vi "Auto.vi"() -> ()   [LabVIEW 2020]
uses:
  Global_Variable/A180648.vi
  Global_Variable/Global.vi
  Global_Variable/System_Conf.vi
  <userlib>/_MGI/1D Array/MGI Running Average/MGI Running Average(SGL).vi
  <userlib>/_MGI/1D Array/MGI Running Average/MGI Running Average(DBL).vi
  Libraries/S7/S7.lvlib
panel:
  out "磨合正向初始化":bool
  out "磨合逆向初始化":bool
  out "试验项_Event":refnum<user-event>
  out "产品_EVENT":refnum<user-event>
  out "布尔":bool=TRUE
  out "T1+T2":dbl
  out "T2":dbl
  out "T1":dbl
  out "吸收电流":sgl
  out "输出扭矩(大)":sgl
  out "输入扭矩":sgl
  out "力特性逆向去程":bool
  out "力特性正向去程":bool
  out "力特性逆向回程":bool
  out "力特性正向回程":bool
  out "逆向空载正向初始化":bool
  out "逆向空载逆向初始化":bool
  out "功能正向初始化":bool
  out "功能逆向初始化":bool
  out "空载逆向初始化":bool
  out "空载正向初始化":bool
  out "当前车速":i32
  out "试验项目":T1(tab)
  out "空载试验":cluster{dbl[], dbl[]}[](graph)
  out "功能试验":cluster{dbl[], dbl[]}[](graph)
  out "力特性试验":cluster{dbl[], dbl[]}[](graph)
  out "电流特性试验":cluster{dbl[], dbl[]}[](graph)
  out "传感器特性试验":cluster{dbl[], dbl[]}[](graph)
  out "逆向空载试验":cluster{dbl[], dbl[]}[](graph)
  out "磨合":cluster{dbl[], dbl[]}[](graph)
  out "振动2NHV-FFT":cluster{"f0":dbl, "df":dbl, "magnitude":dbl[]}[](graph)
  out "振动1NVH-FFT":cluster{"f0":dbl, "df":dbl, "magnitude":dbl[]}[](graph)
  in  "判定结果":bool[][](array[boolean])=[[TRUE]]
  in  "STEP":string
  # "车速0"
  # "车速1"
  # "车速2"
  # "车速3"
  # "车速4"
  # "车速5"
  # "车速0"
  # "车速1"
  # "车速2"
  # "车速3"
  # "车速4"
  # "车速5"
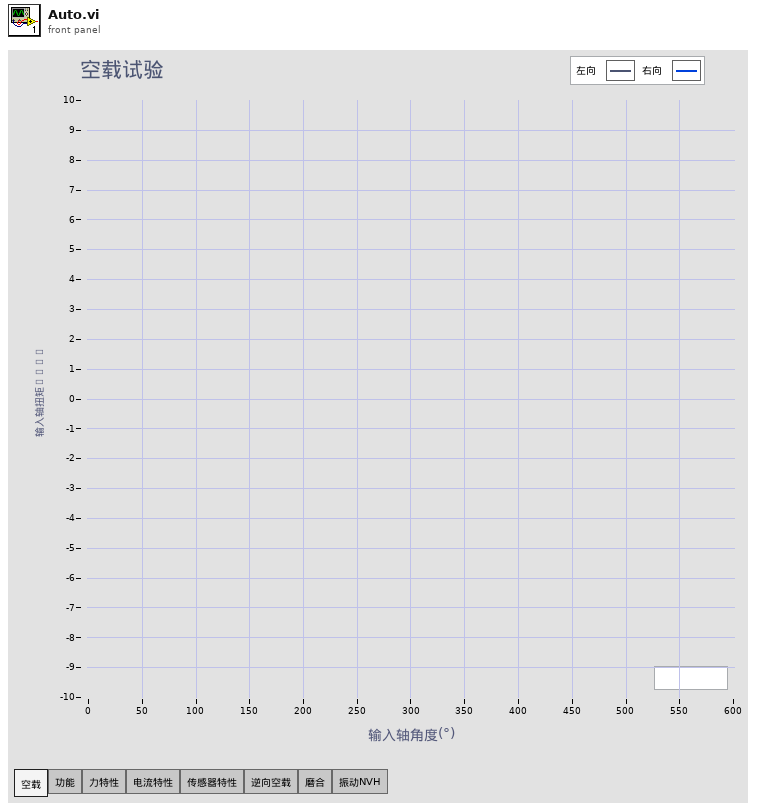
[diagram p1: front panel]
types:
  T1 = enum32{"空载", "功能", "力特性", "电流特性", "传感器特性", "逆向空载", "磨合", "振动NVH"}
  T2 = enum32{"Invalid", "Standard", "Closed", "Hidden", "Minimized", "Maximized"}
  T3 = cluster{"输入轴扭矩":dbl, "输出轴扭矩小量程":dbl, "输出轴扭矩大量程":dbl}
  T4 = enum32{"空载", "功能", "力特性", "电流特性", "传感器特性", "逆向空载", "振动NVH", "磨合", "完成"}
  T5 = enum16{"Left Button", "Center Button", "Right Button", "Window Close"}
  T6 = enum16{"角度标定状态", "角度标定", "角度标定清除", "扭矩标定状态", "扭矩标定", "扭矩标定清除", "内部软件版本号", "客户软件版本号"}
  T7 = typedef "System_conf.ctl" = cluster{"空载滤波":bool, "逆向空载滤波":bool, "空载扭矩系数":dbl, "逆向空载扭矩系数":dbl}
  T8 = enum32{"Bad", "Idle", "Run top level", "Running"}
  T9 = cluster{"扭矩判定范围":cluster{"单位":string, "下限":dbl, "上限":dbl}, "正向扭矩最大值":cluster{"单位":string, "下限":dbl, "上限":dbl}, "正向扭矩最小值":cluster{"单位":string, "下限":dbl, "上限":dbl}, "正向扭矩平均值":cluster{"单位":string, "下限":dbl, "上限":dbl}, "正向扭矩波动值":cluster{"单位":string, "下限":dbl, "上限":dbl}, "逆向扭矩最大值":cluster{"单位":string, "下限":dbl, "上限":dbl}, "逆向扭矩最小值":cluster{"单位":string, "下限":dbl, "上限":dbl}, "逆向扭矩平均值":cluster{"单位":string, "下限":dbl, "上限":dbl}, "逆向扭矩波动值":cluster{"单位":string, "下限":dbl, "上限":dbl}, "正逆向扭矩差值":cluster{"单位":string, "下限":dbl, "上限":dbl}, "启动力矩":cluster{"单位":string, "下限":dbl, "上限":dbl}}
  T10 = cluster{"扭矩判定范围":cluster{"单位":string, "下限":dbl, "上限":dbl}, "正向扭矩最大值":cluster{"单位":string, "下限":dbl, "上限":dbl}, "正向扭矩最小值":cluster{"单位":string, "下限":dbl, "上限":dbl}, "正向扭矩平均值":cluster{"单位":string, "下限":dbl, "上限":dbl}, "正向扭矩波动值":cluster{"单位":string, "下限":dbl, "上限":dbl}, "逆向扭矩最大值":cluster{"单位":string, "下限":dbl, "上限":dbl}, "逆向扭矩最小值":cluster{"单位":string, "下限":dbl, "上限":dbl}, "逆向扭矩平均值":cluster{"单位":string, "下限":dbl, "上限":dbl}, "逆向扭矩波动值":cluster{"单位":string, "下限":dbl, "上限":dbl}, "正逆向扭矩差值":cluster{"单位":string, "下限":dbl, "上限":dbl}}
  T11 = cluster{"对称性检测点":cluster{"单位":string, "下限":dbl, "上限":dbl}, "对称度":cluster{"单位":string, "下限":dbl, "上限":dbl}, "目标输出扭矩1":cluster{"单位":string, "下限":dbl, "上限":dbl}, "目标1正向输入扭矩":cluster{"单位":string, "下限":dbl, "上限":dbl}, "目标1逆向输入扭矩":cluster{"单位":string, "下限":dbl, "上限":dbl}, "目标1正逆向扭矩差":cluster{"单位":string, "下限":dbl, "上限":dbl}, "目标1输入扭矩滞后":cluster{"单位":string, "下限":dbl, "上限":dbl}, "目标输出扭矩2":cluster{"单位":string, "下限":dbl, "上限":dbl}, "目标2正向输入扭矩":cluster{"单位":string, "下限":dbl, "上限":dbl}, "目标2逆向输入扭矩":cluster{"单位":string, "下限":dbl, "上限":dbl}, "目标2正逆向扭矩差":cluster{"单位":string, "下限":dbl, "上限":dbl}, "目标2输入扭矩滞后":cluster{"单位":string, "下限":dbl, "上限":dbl}, "目标输出扭矩3":cluster{"单位":string, "下限":dbl, "上限":dbl}, "目标3正向输入扭矩":cluster{"单位":string, "下限":dbl, "上限":dbl}, "目标3逆向输入扭矩":cluster{"单位":string, "下限":dbl, "上限":dbl}, "目标3正逆向扭矩差":cluster{"单位":string, "下限":dbl, "上限":dbl}, "目标3输入扭矩滞后":cluster{"单位":string, "下限":dbl, "上限":dbl}, "目标输出扭矩4":cluster{"单位":string, "下限":dbl, "上限":dbl}, "目标4正向输入扭矩":cluster{"单位":string, "下限":dbl, "上限":dbl}, "目标4逆向输入扭矩":cluster{"单位":string, "下限":dbl, "上限":dbl}, "目标4正逆向扭矩差":cluster{"单位":string, "下限":dbl, "上限":dbl}, "目标4输入扭矩滞后":cluster{"单位":string, "下限":dbl, "上限":dbl}, "目标输出扭矩5":cluster{"单位":string, "下限":dbl, "上限":dbl}, "目标5正向输入扭矩":cluster{"单位":string, "下限":dbl, "上限":dbl}, "目标5逆向输入扭矩":cluster{"单位":string, "下限":dbl, "上限":dbl}, "目标5正逆向扭矩差":cluster{"单位":string, "下限":dbl, "上限":dbl}, "目标5输入扭矩滞后":cluster{"单位":string, "下限":dbl, "上限":dbl}}[]
  T12 = cluster{"主副信号和MAX":cluster{"单位":string, "下限":dbl, "上限":dbl}, "主副信号和MIN":cluster{"单位":string, "下限":dbl, "上限":dbl}, "主信号线性误差":cluster{"单位":string, "下限":dbl, "上限":dbl}, "副信号线性误差":cluster{"单位":string, "下限":dbl, "上限":dbl}, "主信号MAX":cluster{"单位":string, "下限":dbl, "上限":dbl}, "主信号MIN":cluster{"单位":string, "下限":dbl, "上限":dbl}, "副信号MAX":cluster{"单位":string, "下限":dbl, "上限":dbl}, "副信号MIN":cluster{"单位":string, "下限":dbl, "上限":dbl}, "中心偏移量":cluster{"单位":string, "下限":dbl, "上限":dbl}, "定点设置":cluster{"单位":string, "下限":dbl, "上限":dbl}, "定点左侧主信号":cluster{"单位":string, "下限":dbl, "上限":dbl}, "定点左侧副信号":cluster{"单位":string, "下限":dbl, "上限":dbl}, "定点右侧主信号":cluster{"单位":string, "下限":dbl, "上限":dbl}, "定点右侧副信号":cluster{"单位":string, "下限":dbl, "上限":dbl}}
  T13 = cluster{"对称性检测点":cluster{"单位":string, "下限":dbl, "上限":dbl}, "对称度":cluster{"单位":string, "下限":dbl, "上限":dbl}, "最大电流":cluster{"单位":string, "下限":dbl, "上限":dbl}, "目标输出电流1":cluster{"单位":string, "下限":dbl, "上限":dbl}, "目标1正向输入扭矩":cluster{"单位":string, "下限":dbl, "上限":dbl}, "目标1逆向输入扭矩":cluster{"单位":string, "下限":dbl, "上限":dbl}, "目标1正逆向扭矩差":cluster{"单位":string, "下限":dbl, "上限":dbl}, "目标1输入扭矩滞后":cluster{"单位":string, "下限":dbl, "上限":dbl}, "目标输出电流2":cluster{"单位":string, "下限":dbl, "上限":dbl}, "目标2正向输入扭矩":cluster{"单位":string, "下限":dbl, "上限":dbl}, "目标2逆向输入扭矩":cluster{"单位":string, "下限":dbl, "上限":dbl}, "目标2正逆向扭矩差":cluster{"单位":string, "下限":dbl, "上限":dbl}, "目标2输入扭矩滞后":cluster{"单位":string, "下限":dbl, "上限":dbl}, "目标输出电流3":cluster{"单位":string, "下限":dbl, "上限":dbl}, "目标3正向输入扭矩":cluster{"单位":string, "下限":dbl, "上限":dbl}, "目标3逆向输入扭矩":cluster{"单位":string, "下限":dbl, "上限":dbl}, "目标3正逆向扭矩差":cluster{"单位":string, "下限":dbl, "上限":dbl}, "目标3输入扭矩滞后":cluster{"单位":string, "下限":dbl, "上限":dbl}, "目标输出电流4":cluster{"单位":string, "下限":dbl, "上限":dbl}, "目标4正向输入扭矩":cluster{"单位":string, "下限":dbl, "上限":dbl}, "目标4逆向输入扭矩":cluster{"单位":string, "下限":dbl, "上限":dbl}, "目标4正逆向扭矩差":cluster{"单位":string, "下限":dbl, "上限":dbl}, "目标4输入扭矩滞后":cluster{"单位":string, "下限":dbl, "上限":dbl}, "目标输出电流5":cluster{"单位":string, "下限":dbl, "上限":dbl}, "目标5正向输入扭矩":cluster{"单位":string, "下限":dbl, "上限":dbl}, "目标5逆向输入扭矩":cluster{"单位":string, "下限":dbl, "上限":dbl}, "目标5正逆向扭矩差":cluster{"单位":string, "下限":dbl, "上限":dbl}, "目标5输入扭矩滞后":cluster{"单位":string, "下限":dbl, "上限":dbl}}[]
  T14 = cluster{"振动1频率检测段1范围":cluster{"单位":string, "下限":dbl, "上限":dbl}, "振动1频率检测段2范围":cluster{"单位":string, "下限":dbl, "上限":dbl}, "振动1频率检测段3范围":cluster{"单位":string, "下限":dbl, "上限":dbl}, "振动1频率检测段4范围":cluster{"单位":string, "下限":dbl, "上限":dbl}, "振动1频率检测段5范围":cluster{"单位":string, "下限":dbl, "上限":dbl}, "振动2频率检测段1范围":cluster{"单位":string, "下限":dbl, "上限":dbl}, "振动2频率检测段2范围":cluster{"单位":string, "下限":dbl, "上限":dbl}, "振动2频率检测段3范围":cluster{"单位":string, "下限":dbl, "上限":dbl}, "振动2频率检测段4范围":cluster{"单位":string, "下限":dbl, "上限":dbl}, "振动2频率检测段5范围":cluster{"单位":string, "下限":dbl, "上限":dbl}}
  T15 = cluster{"振动1频率检测段1振幅":cluster{"单位":string, "下限":dbl, "上限":dbl}, "振动1频率检测段2振幅":cluster{"单位":string, "下限":dbl, "上限":dbl}, "振动1频率检测段3振幅":cluster{"单位":string, "下限":dbl, "上限":dbl}, "振动1频率检测段4振幅":cluster{"单位":string, "下限":dbl, "上限":dbl}, "振动1频率检测段5振幅":cluster{"单位":string, "下限":dbl, "上限":dbl}, "振动2频率检测段1振幅":cluster{"单位":string, "下限":dbl, "上限":dbl}, "振动2频率检测段2振幅":cluster{"单位":string, "下限":dbl, "上限":dbl}, "振动2频率检测段3振幅":cluster{"单位":string, "下限":dbl, "上限":dbl}, "振动2频率检测段4振幅":cluster{"单位":string, "下限":dbl, "上限":dbl}, "振动2频率检测段5振幅":cluster{"单位":string, "下限":dbl, "上限":dbl}}
  T16 = cluster{"扭矩判定范围":cluster{"单位":string, "下限":dbl, "上限":dbl}, "正向扭矩最大值":cluster{"单位":string, "下限":dbl, "上限":dbl}, "正向扭矩最小值":cluster{"单位":string, "下限":dbl, "上限":dbl}, "正向扭矩平均值":cluster{"单位":string, "下限":dbl, "上限":dbl}, "正向扭矩波动值":cluster{"单位":string, "下限":dbl, "上限":dbl}, "逆向扭矩最大值":cluster{"单位":string, "下限":dbl, "上限":dbl}, "逆向扭矩最小值":cluster{"单位":string, "下限":dbl, "上限":dbl}, "逆向扭矩平均值":cluster{"单位":string, "下限":dbl, "上限":dbl}, "逆向扭矩波动值":cluster{"单位":string, "下限":dbl, "上限":dbl}, "正逆向扭矩差值":cluster{"单位":string, "下限":dbl, "上限":dbl}, "启动扭矩范围":cluster{"单位":string, "下限":dbl, "上限":dbl}, "启动扭矩":cluster{"单位":string, "下限":dbl, "上限":dbl}}
  T17 = cluster{"试验速度":dbl, "试验角度":dbl, "负载扭矩":dbl, "保护扭矩":dbl}
  T18 = cluster{"输入旋转位移":sgl, "输入移载位移":sgl, "工装移载位移":sgl, "输入编码位移":sgl, "输入扭矩":sgl, "输出扭矩(小)":sgl, "输出扭矩(大)":sgl, "吸收电流":sgl, "Factorysensor":sgl, "输出轴旋转角度":sgl, "输出轴移栽位移":sgl, "Factorysensor2":sgl}
  T19 = typedef "svc_Spectrum Info.ctl" = cluster{"channel name":string, "description":string, "x-axis units":T20, "spectral info":cluster{"spectrum type":T21, "linear/dB":enum16{"linear", "dB"}, "window":u16, "window size":i32, "FFT size":i32}, "engineering units":T22, "custom label":string, "dB reference [EU]":dbl, "peak units":enum16{"rms", "peak", "peak-peak"}, "weighting filter":T23, "spectral density?":bool, "unit label":string, "spectrum skewed?":bool, "complimentary spectrum units":T24}
  T20 = typedef "svc_X-Axis Units.ctl" = u16
  T21 = typedef "svc_Spectrum Type.ctl" = enum16{"FFT Spectrum [complex]", "Amplitude [Magnitude]", "Power [Magnitude^2]", "Cross Spectrum [complex]", "Frequency Response [Complex]"}
  T22 = typedef "svc_Engineering Units Text Ring.ctl" = u16
  T23 = typedef "svc_Weighting Filter Text Ring.ctl" = u16
  T24 = typedef "svc_Complimentary Spectrum Units.ctl" = enum16{"none", "radians", "degrees", "cycles", "imaginary"}
  T25 = typedef "lveventtype.ctl" = enum32{"Null", "Timeout", "Annotation Menu Selection", "Annotation Menu Selection?", "App Instance Close", "App Instance Close?", "Autoscale Range Change", "Bookmark Info Change", "Cell Edit", "Cell Edit?", "Cursor Grab", "Cursor Grab?", "Cursor Menu Selection", "Cursor Menu Selection?", "Cursor Move", "Cursor Release", "Data Change", "Direction Change", "Display State Change", "Drag Ended", "Drag Enter", "Drag Leave", "Drag Over", "Drag Source Update", "Drag Starting", "Drag Starting?", "Drop", "Exec State Change", "Key Down", "Key Down?", "Key Repeat", "Key Repeat?", "Key Up", "Listbox Double Click", "Menu Activation?", "Menu Selection (App)", "Menu Selection? (App)", "Menu Selection (User)", "Mouse Down", "Mouse Down?", "Mouse Enter", "Mouse Leave", "Mouse Move", "Mouse Up", "Mouse Wheel", "NI Security User Change (App)", "Pane Size", "Panel Close", "Panel Close?", "Panel Resize", "Plot Attribute Change", "Scale Range Change", "Shortcut Menu Activation?", "Shortcut Menu Selection (App)", "Shortcut Menu Selection? (App)", "Shortcut Menu Selection (User)", "Tree Double Click", "Tree Drag", "Tree Drag?", "Tree Drop", "Tree Drop?", "Tree Item Close", "Tree Item Close?", "Tree Item Open", "Tree Item Open?", "User Event", "Value Change"}
  T26 = typedef "LVPoint32TypeDef.ctl" = cluster{"Horizontal":i32, "Vertical":i32}
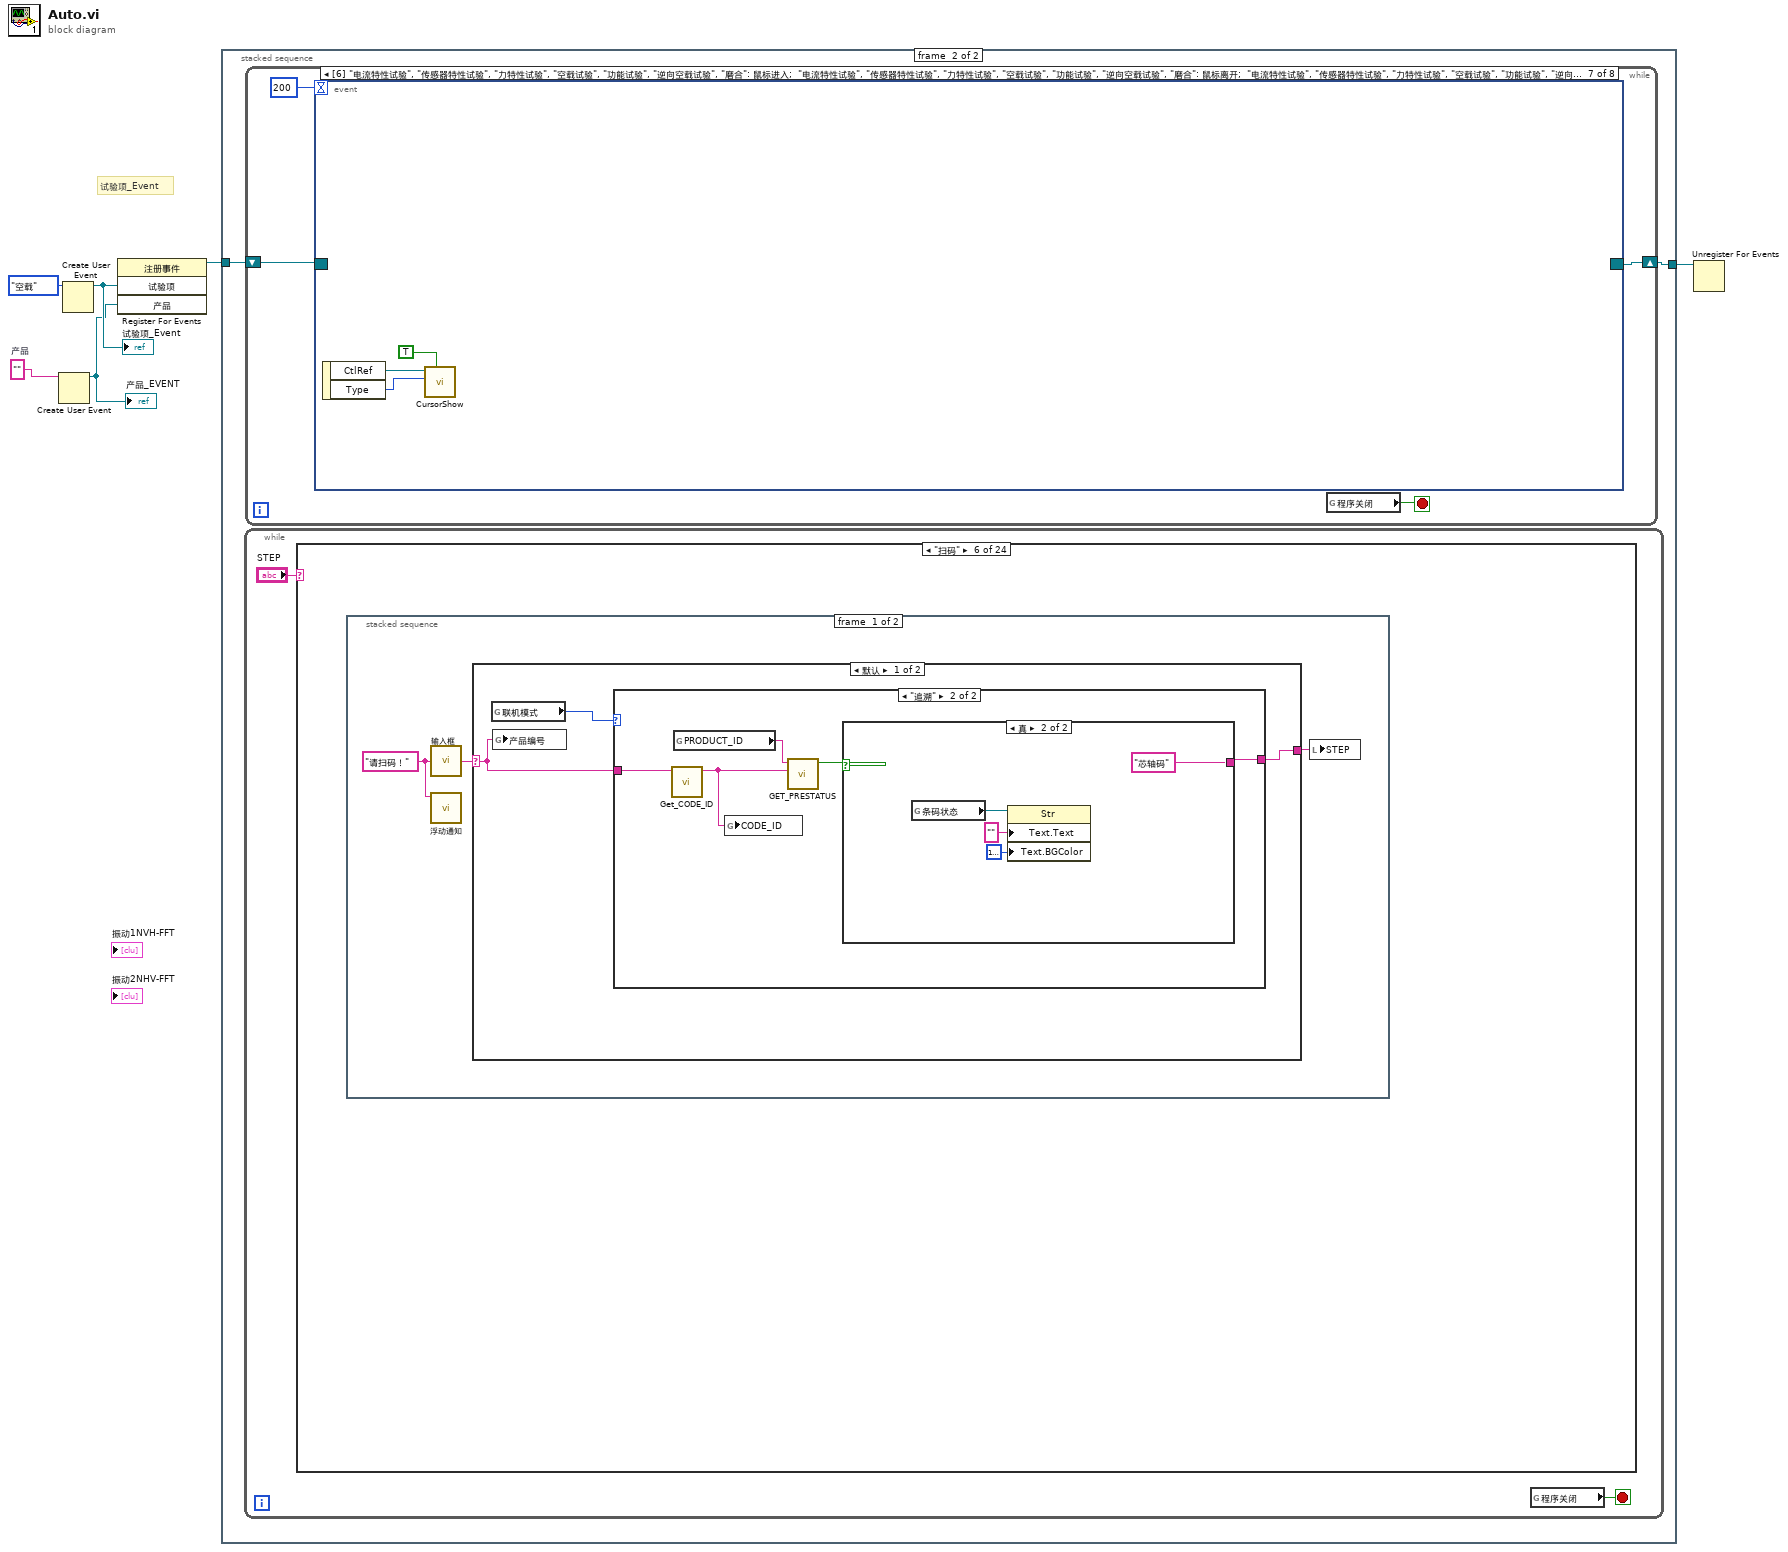
[diagram p0: block diagram]
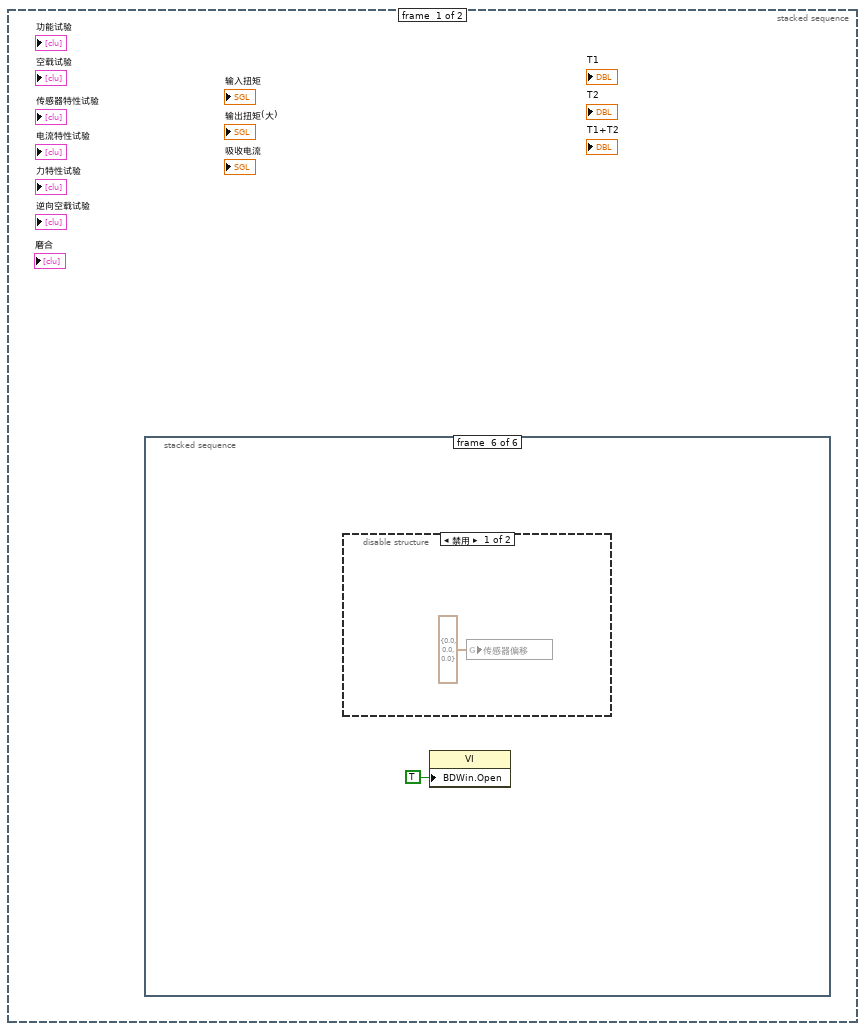
[diagram p2: hidden frame]
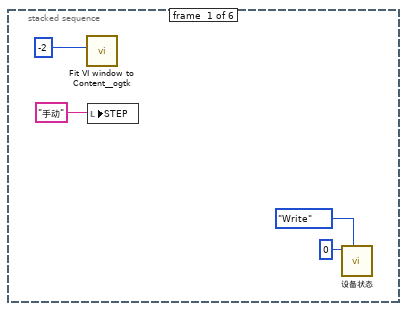
[diagram p3: hidden frame]
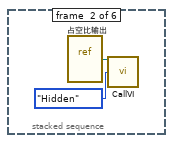
[diagram p4: hidden frame]
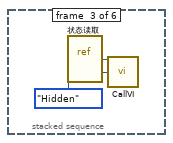
[diagram p5: hidden frame]
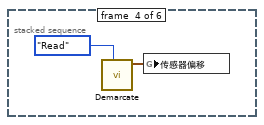
[diagram p6: hidden frame]
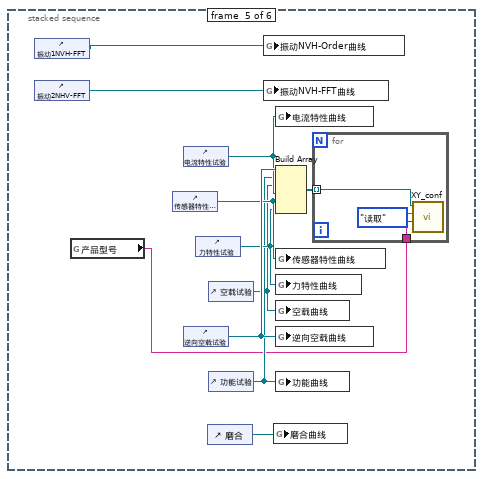
[diagram p7: hidden frame]
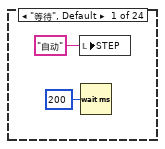
[diagram p9: hidden frame]
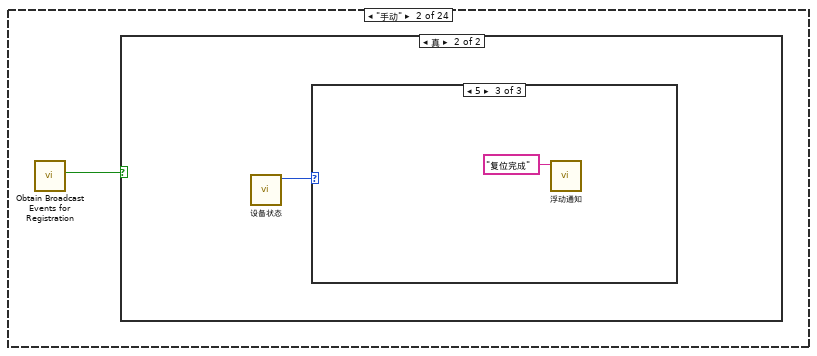
[diagram p10: hidden frame]
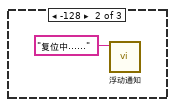
[diagram p13: hidden frame]
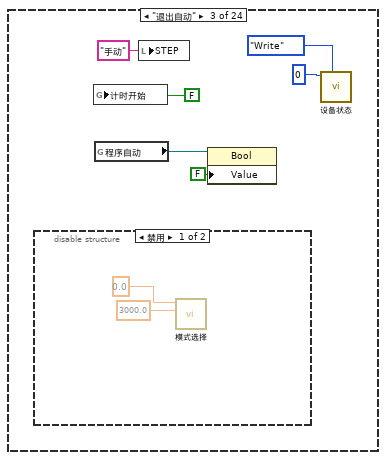
[diagram p14: hidden frame]
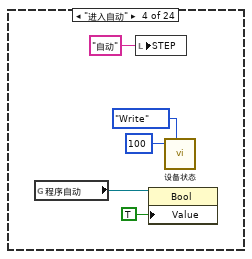
[diagram p16: hidden frame]
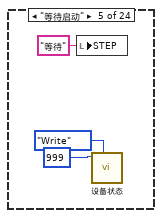
[diagram p17: hidden frame]
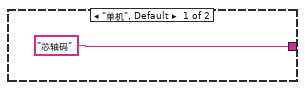
[diagram p18: hidden frame]
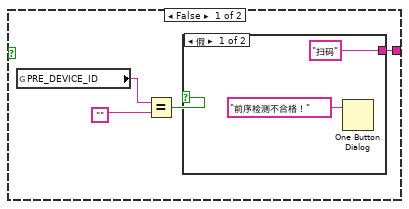
[diagram p19: hidden frame]
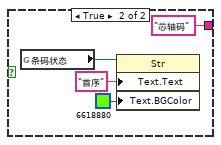
[diagram p20: hidden frame]
diagram:
  w2 = ""  # 产品
  # "试验项_Event"
  n1 = Create User Event(user event datatype=w2) -> (user event=w1:refnum<user-event>)  [unwired: 1 in, 1 out]
  "产品_EVENT" <- w1
  n2 = Create User Event(user event datatype=T1."空载" ("试验项")) -> (user event=w4:refnum<user-event>)  [unwired: 1 in, 1 out]
  "试验项_Event" <- w4
  n3 = register-events(w4, w1) -> (reference out=w5:refnum<event-registration>)  [unwired: 2 in, 1 out]
  n4 = stacked-sequence {
    tunnel: w5 -> [_ w34]
    tunnel: [_ w33] -> w3
    frame #0 {
      n5 = stacked-sequence {
        frame #0 {
          n6 = call <userlib>:"Fit VI window to Content__ogtk.vi"("border spacing (2 px)"=-2) -> ()  [unwired: 5 in, 2 out]
          n7 = local write "STEP"("手动" ("STEP")) -> ()
          n8 = call "设备状态.vi"("枚举"=enum16{"Read", "Write"}."Write", "Status_Write"=i16 0) -> ()  [unwired: 9 in, 1 out]
        }
        frame #1 {
          n9 = vi-ref "占空比输出.vi"() -> (w12:refnum<vi>)
          n10 = call "CallVI.vi"("VI引用"=w12, "状态"=T2."Hidden") -> ()  [unwired: 12 in, 2 out]
        }
        frame #2 {
          n11 = vi-ref "状态读取.vi"() -> (w14:refnum<vi>)
          n12 = call "CallVI.vi"("VI引用"=w14, "状态"=T2."Hidden") -> ()  [unwired: 12 in, 2 out]
        }
        frame #3 {
          n13 = call "Demarcate.vi"("Mode"=enum16{"Read", "Write"}."Read") -> ("Sensor OUT"=w16:T3)  [unwired: 9 in, 1 out]
          n14 = global write "传感器偏移.vi" "传感器偏移"(w16) -> ()
        }
        frame #4 {
          n15 = control-ref of="振动1NVH-FFT"() -> (w20:refnum<vi>)
          n16 = control-ref of="振动2NHV-FFT"() -> (w19:refnum<vi>)
          n17 = global read "Global.vi" "产品型号"() -> (w18:string)
          n18 = control-ref of="传感器特性试验"() -> (w25:refnum<vi>)
          n19 = control-ref of="电流特性试验"() -> (w26:refnum<vi>)
          n20 = control-ref of="逆向空载试验"() -> (w27:refnum<vi>)
          n21 = control-ref of="力特性试验"() -> (w24:refnum<vi>)
          n22 = control-ref of="磨合"() -> (w17:refnum<vi>)
          n23 = control-ref of="空载试验"() -> (w22:refnum<vi>)
          n24 = control-ref of="功能试验"() -> (w23:refnum<vi>)
          n25 = global write "A180648.vi" "振动NVH-Order曲线"(w20) -> ()
          n26 = global write "A180648.vi" "振动NVH-FFT曲线"(w19) -> ()
          n27 = global write "A180648.vi" "磨合曲线"(w17) -> ()
          n28 = global write "A180648.vi" "电流特性曲线"(w26) -> ()
          n29 = Build Array(w27, w23, w22, w26, w25, w24) -> (w21:refnum<vi>[])
          n30 = global write "A180648.vi" "传感器特性曲线"(w25) -> ()
          n31 = global write "A180648.vi" "力特性曲线"(w24) -> ()
          n32 = global write "A180648.vi" "空载曲线"(w22) -> ()
          n33 = global write "A180648.vi" "逆向空载曲线"(w27) -> ()
          n34 = global write "A180648.vi" "功能曲线"(w23) -> ()
          n35 = for {
            tunnel: w21 -> [w29] mode=indexing
            tunnel: w18 -> [w28]
            n36 = call "XY_conf.vi"("方式"=enum16{"写入", "读取"}."读取", "产品"=w28, "XY图引用"=w29) -> ()  [unwired: 4 in, 1 out]
          }
        }
        frame #5 {
          n37 = disable-structure shown="禁用" {
            frame Disabled {
              n38 = global write "传感器偏移.vi" "传感器偏移"(T3 {"输入轴扭矩"=0.0, "输出轴扭矩小量程"=0.0, "输出轴扭矩大量程"=0.0} ("传感器偏移")) -> ()
            }
            frame Enabled {
            }
          }
          n39 = property class="VI"("BDWin.Open"=TRUE ("程序框图窗口:打开")) -> ()  [unwired: 2 in, 2 out]
        }
      }
    }
    frame #1 {
      n40 = while {
        stop <- w36 stop-if-true
        n41 = case shown="\"扫码\"" "STEP" {
          frame "等待", Default {
            n42 = local write "STEP"("自动" ("STEP")) -> ()
            n43 = Wait (ms)(milliseconds to wait=u32 200 ("等待时间（毫秒）")) -> ()  [unwired: 1 out]
          }
          frame "手动" {
            n44 = call "Obtain Broadcast Events for Registration.vi"() -> ("Already running?"=w39:bool)  [unwired: 9 in, 2 out]
            n45 = case shown="真" w39 {
              frame False {
              }
              frame True {
                n46 = call "设备状态.vi"() -> ("Status_Read"=w40:i16)  [unwired: 11 in]
                n47 = case shown="5" w40 {
                  frame 0, Default {
                  }
                  frame -128 {
                    n48 = call "浮动通知.vi"("通知内容"="复位中……" ("Status")) -> ()  [unwired: 11 in]
                  }
                  frame 5 {
                    n49 = call "浮动通知.vi"("通知内容"="复位完成" ("Status")) -> ()  [unwired: 11 in]
                  }
                }
              }
            }
          }
          frame "退出自动" {
            n50 = disable-structure shown="禁用" {
              frame Disabled {
                n51 = call-poly "模式选择.vi"("Max Torque"=sgl 3000.0, "Velocity"=sgl 0.0) -> ()  [unwired: 9 in, 1 out]
              }
              frame Enabled {
              }
            }
            n52 = global write "Global.vi" "计时开始"(FALSE ("计时开始")) -> ()
            n53 = global read "Global.vi" "程序自动"() -> (w46:refnum<vi>)
            n54 = local write "STEP"("手动" ("STEP")) -> ()
            n55 = property class="Bool"(reference=w46, "Value"=FALSE) -> ()  [unwired: 1 in, 2 out]
            n56 = call "设备状态.vi"("枚举"=enum16{"Read", "Write"}."Write", "Status_Write"=i16 0) -> ()  [unwired: 9 in, 1 out]
          }
          frame "进入自动" {
            n57 = global read "Global.vi" "程序自动"() -> (w52:refnum<vi>)
            n58 = local write "STEP"("自动" ("STEP")) -> ()
            n59 = property class="Bool"(reference=w52, "Value"=TRUE) -> ()  [unwired: 1 in, 2 out]
            n60 = call "设备状态.vi"("枚举"=enum16{"Read", "Write"}."Write", "Status_Write"=i16 100) -> ()  [unwired: 9 in, 1 out]
          }
          frame "等待启动" {
            n61 = local write "STEP"("等待" ("STEP")) -> ()
            n62 = call "设备状态.vi"("枚举"=enum16{"Read", "Write"}."Write", "Status_Write"=i16 999) -> ()  [unwired: 9 in, 1 out]
          }
          frame "扫码" {
            n63 = stacked-sequence {
              frame #0 {
                w60 = "请扫码！" ("提示信息")
                n64 = call "输入框.vi"("提示信息"=w60) -> ("条形码输出"=w61:string)
                n65 = call "浮动通知.vi"("通知内容"=w60) -> ()  [unwired: 11 in]
                n66 = case shown="默认" w61 {
                  selector: w61 -> [w63 _]
                  tunnel: [w64 "退出自动" ("State(s) in Front (\"\")")] -> w59
                  frame Default {
                    n67 = global read "Global.vi" "联机模式"() -> (w62:enum16{"单机", "追溯"})
                    n68 = global write "Global.vi" "产品编号"(w63) -> ()
                    n69 = case shown="\"追溯\"" w62 {
                      tunnel: ["芯轴码" ("State(s) in Front (\"\")") w70] -> w64
                      tunnel: w63 -> [_ w67]
                      frame "单机", Default {
                      }
                      frame "追溯" {
                        n70 = call "Get_CODE_ID.vi"("CODE_MAIN"=w67) -> ("CODE_ID"=w66:string)  [unwired: 10 in]
                        n71 = global read "追溯Global.vi" "PRODUCT_ID"() -> (w69:string)
                        n72 = global write "追溯Global.vi" "CODE_ID"(w66) -> ()
                        n73 = call "GET_PRESTATUS.vi"("CODE_ID"=w66, "PRODUCT_ID"=w69) -> ("OK?"=w68:bool)  [unwired: 9 in]
                        n74 = case shown="真" w68 {
                          tunnel: [w74 "芯轴码" ("State(s) in Front (\"\")")] -> w70
                          frame False {
                            n75 = global read "追溯Global.vi" "PRE_DEVICE_ID"() -> (w73:string)
                            n76 = Equal?(x=w73, y="") -> (x = y?=w71:bool)
                            n77 = case shown="假" w71 {
                              tunnel: ["扫码" ("State(s) in Front (\"\")") "芯轴码" ("State(s) in Front (\"\")")] -> w74
                              frame False {
                                n78 = One Button Dialog(message="前序检测不合格！" ("消息")) -> ()  [unwired: 1 in, 1 out]
                              }
                              frame True {
                                n79 = global read "Global.vi" "条码状态"() -> (w79:refnum<vi>)
                                n80 = property class="Str"(reference=w79, "Text.Text"="首序" ("文本.文本"), "Text.BGColor"=u32 6618880 ("文本.文本颜色:背景色")) -> ()  [unwired: 1 in, 2 out]
                              }
                            }
                          }
                          frame True {
                            n81 = global read "Global.vi" "条码状态"() -> (w83:refnum<vi>)
                            n82 = property class="Str"(reference=w83, "Text.Text"="" ("文本.文本"), "Text.BGColor"=u32 16777216 ("文本.文本颜色:背景色")) -> ()  [unwired: 1 in, 2 out]
                          }
                        }
                      }
                    }
                  }
                  frame "", "exit" {
                  }
                }
                n83 = local write "STEP"(w59) -> ()
              }
              frame #1 {
                n84 = Wait (ms)(milliseconds to wait=u32 200 ("等待时间（毫秒）")) -> ()  [unwired: 1 out]
              }
            }
          }
          frame "芯轴码" {
            n85 = stacked-sequence {
              frame #0 {
                w88 = "请扫芯轴码！" ("提示信息")
                n86 = call "输入框.vi"("提示信息"=w88) -> ("条形码输出"=w89:string)
                n87 = call "浮动通知.vi"("通知内容"=w88) -> ()  [unwired: 11 in]
                n88 = case shown="默认" w89 {
                  selector: w89 -> [w91 _]
                  tunnel: [w92 "退出自动" ("State(s) in Front (\"\")")] -> w87
                  frame Default {
                    n89 = global read "Global.vi" "联机模式"() -> (w90:enum16{"单机", "追溯"})
                    n90 = global write "Global.vi" "芯轴码"(w91) -> ()
                    n91 = case shown="\"追溯\"" w90 {
                      tunnel: ["等待启动" ("State(s) in Front (\"\")") w98] -> w92
                      tunnel: w91 -> [_ w94]
                      frame "单机", Default {
                      }
                      frame "追溯" {
                        n92 = global read "Global.vi" "产品编号"() -> (w97:string)
                        n93 = call "Get_SENSOR.vi"("CODE_MAIN"=w97) -> ("CODE_SENSOR"=w95:string)  [unwired: 10 in]
                        n94 = Equal?(x=w95, y=w94) -> (x = y?=w96:bool)
                        n95 = case shown="真" w96 {
                          tunnel: ["芯轴码" ("State(s) in Front (\"\")") "等待启动" ("State(s) in Front (\"\")")] -> w98
                          frame False {
                            n96 = One Button Dialog(message="壳体码与芯轴码不匹配！" ("消息")) -> ()  [unwired: 1 in, 1 out]
                          }
                          frame True {
                            n97 = global read "Global.vi" "生产数量"() -> (w101:i32)
                            n98 = Increment(x=w101) -> (x+1=w102:i32)
                            n99 = global write "Global.vi" "生产数量"(w102) -> ()
                          }
                        }
                      }
                    }
                  }
                  frame "", "exit" {
                  }
                }
                n100 = local write "STEP"(w87) -> ()
              }
              frame #1 {
                n101 = Wait (ms)(milliseconds to wait=u32 200 ("等待时间（毫秒）")) -> ()  [unwired: 1 out]
              }
            }
          }
          frame "初始化" {
            n102 = stacked-sequence {
              frame #0 {
                w107 = enum16{"Read", "Write"}."Read" ("Mode")
                n103 = global read "Global.vi" "产品型号"() -> (w108:string)
                n104 = global write "Global.vi" "IO_Stop"(TRUE ("IO_Stop")) -> ()
                n105 = global write "Global.vi" "计时开始"(TRUE ("计时开始")) -> ()
                n106 = local write "判定结果"(bool[][] [] ("判定结果")) -> ()
                n107 = call "Demarcate.vi"("Mode"=w107, "Section"=w108) -> ("Sensor OUT"=w106:T3)  [unwired: 8 in, 1 out]
                n108 = call "System_Conf_RW.vi"("Mode"=w107, "Section"=w108) -> ("system_out"=w110:T7)  [unwired: 8 in, 1 out]
                n109 = global write "A180648.vi" "当前车速"(u16 0 ("当前车速")) -> ()
                n110 = global write "System_Conf.vi" "system"(w110) -> ()
                n111 = global write "传感器偏移.vi" "传感器偏移"(w106) -> ()
                "当前车速" <- 0 ("当前车速")
              }
              frame #1 {
                w115 = TRUE
                "逆向空载正向初始化" <- w115
                "逆向空载逆向初始化" <- w115
                "空载正向初始化" <- w115
                "空载逆向初始化" <- w115
                "功能正向初始化" <- w115
                "功能逆向初始化" <- w115
                "力特性逆向去程" <- w115
                "力特性正向去程" <- w115
                "力特性逆向回程" <- w115
                "力特性正向回程" <- w115
                "磨合正向初始化" <- w115
                "磨合逆向初始化" <- w115
              }
              frame #2 {
                n112 = for {
                  N: 24 -> [_]
                  tunnel: [cluster{dbl[], dbl[]} {[], []}] -> w116 mode=indexing
                  tunnel: [cluster{"f0":dbl, "df":dbl, "magnitude":dbl[]} {"f0"=0.0, "df"=0.0, "magnitude"=[]} ("power spectrum [dB EU]")] -> w117 mode=indexing
                }
                n113 = local write "振动2NHV-FFT"(w117) -> ()
                n114 = local write "力特性试验"(w116) -> ()
                n115 = local write "电流特性试验"(w116) -> ()
                n116 = local write "空载试验"(w116) -> ()
                n117 = local write "功能试验"(w116) -> ()
                n118 = local write "传感器特性试验"(w116) -> ()
                n119 = local write "逆向空载试验"(w116) -> ()
                n120 = local write "振动1NVH-FFT"(w117) -> ()
                n121 = local write "磨合"(w116) -> ()
              }
              frame #3 {
                n122 = global read "Global.vi" "Result"() -> (w123:refnum<vi>)
                n123 = property class="Tbl"(reference=w123, "Value"=string[][] []) -> (reference out=w124:refnum<vi>, error out=w125:errorcluster)  [unwired: 1 in]
                n124 = property class="Tbl"(reference=w124, error in=w125, "Row Headers[]"=string[] [] ("列首字符串[]")) -> ()  [unwired: 2 out]
              }
              frame #4 {
                n125 = global read "A180648.vi" "LED-传感器特性"() -> (w131:refnum<vi>)
                n126 = global read "A180648.vi" "LED-振动NVH"() -> (w127:refnum<vi>)
                n127 = global read "A180648.vi" "LED-电流特性"() -> (w132:refnum<vi>)
                n128 = global read "A180648.vi" "LED-逆向空载"() -> (w128:refnum<vi>)
                n129 = global read "A180648.vi" "LED-磨合"() -> (w126:refnum<vi>)
                n130 = global read "A180648.vi" "LED-力特性"() -> (w129:refnum<vi>)
                n131 = global read "A180648.vi" "LED-功能"() -> (w134:refnum<vi>)
                n132 = global read "A180648.vi" "LED-空载"() -> (w130:refnum<vi>)
                n133 = Build Array(w131, w132, w134, w130, w129, w128, w127, w126) -> (w133:refnum<vi>[])
                n134 = for {
                  tunnel: w133 -> [w135] mode=indexing
                  n135 = property class="Bool"(reference=w135, "Colors [4]"=cluster{u32, u32}[] [{12369084, 12369084}] ("颜色[4]")) -> ()  [unwired: 1 in, 2 out]
                }
              }
              frame #5 {
                w137 = 1 ("维数大小")
                n136 = Initialize Array(" " ("字符串"), w137, w137, w137) -> (w140:string[][][])
                n137 = global write "A180648.vi" "检测结果"(w140) -> ()
                n138 = global write "A180648.vi" "当前检测项"(T4."空载" ("当前检测项")) -> ()
              }
              frame #6 {
                n139 = global read "Global.vi" "启用CAN"() -> (w144:bool)
                n140 = Select(t="CAN初始化" ("STEP"), s=w144, f="K-Line初始化" ("STEP")) -> (s? t:f=w141:string)
                n141 = local write "STEP"(w141) -> ()
              }
            }
          }
          frame "CAN初始化" {
            n142 = stacked-sequence {
              frame #0 {
                n143 = while {
                  stop <- w145 stop-if-true
                  n144 = vi-ref "CAN.vi"() -> (w150:refnum<vi>)
                  n145 = call "CallVI.vi"("VI引用"=w150, "状态"=T2."Hidden") -> ("VI引用OUT"=w148:refnum<vi>, "错误输出"=w147:errorcluster)  [unwired: 12 in]
                  n146 = property class="VI"(reference=w148, error in=w147) -> ("Exec.State"=w146:T8)  [unwired: 2 out]
                  n147 = case shown="\"Bad\", 默认" w146 {
                    tunnel: [w154 TRUE TRUE] -> w145
                    frame "Bad", Default {
                      n148 = Two Button Dialog(message="CAN卡打开失败！" ("消息"), 1:"重试" ("F按钮名称（“取消”）"), 2:"忽略" ("T按钮名称（“确定”）")) -> (T button?=w154:bool)
                    }
                    frame "Run top level" {
                    }
                    frame "Running" {
                    }
                  }
                }
              }
              frame #1 {
                n149 = while {
                  tunnel: [w159] -> w157
                  i -> [w158]
                  stop <- w160 stop-if-true
                  n150 = global read "Global.vi" "CAN软件版本号"() -> (w162:string)
                  n151 = call "Can软件版本号.vi"() -> ("软件版本号"=w163:string)  [unwired: 11 in]
                  n152 = Equal?(x=w163, y=w162) -> (x = y?=w164:bool)
                  n153 = global write "Global.vi" "软件版本号"(w163) -> ()
                  n154 = case shown="真" w164 {
                    tunnel: w163 -> [w174 _]
                    tunnel: w162 -> [w175 _]
                    tunnel: [w173 T5."Center Button" ("Which Button?")] -> w161
                    tunnel: w158 -> [w172 _]
                    frame False {
                      n155 = Greater Or Equal?(x=w172, y=3) -> (x >= y?=w170:bool)
                      n156 = Format Into String(format string="软件版本号不匹配！\nECU软件版本号：%s\n预期软件版本号：%s" ("格式字符串"), w174, w175) -> (resulting string=w177:string)  [unwired: 2 in, 1 out]
                      n157 = case shown="真" w170 {
                        tunnel: w177 -> [_ w184]
                        tunnel: [T5."Left Button" ("Which Button?") w179] -> w173
                        frame False {
                        }
                        frame True {
                          n158 = call <vilib>:"Three Button Dialog.vi"("Allow user to close window? (TRUE)"=FALSE, "Right Button Text (\"Cancel\")"="取消" ("Right Button Text (\"Cancel\")"), "Center Button Text (\"No\")"="忽略" ("Center Button Text (\"No\")"), "Left Button Text (\"Yes\")"="重试" ("Left Button Text (\"Yes\")"), "message"=w184) -> ("Which Button?"=w179:T5)  [unwired: 6 in]
                        }
                      }
                    }
                    frame True {
                    }
                  }
                  n159 = case shown="\"Center Button\"" w161 {
                    tunnel: [FALSE TRUE TRUE] -> w160
                    tunnel: [_ "角度标定" "退出自动"] -> w159
                    frame "Left Button", Default {
                    }
                    frame "Center Button" {
                    }
                    frame "Right Button" {
                    }
                  }
                }
                n160 = local write "STEP"(w157) -> ()
              }
            }
          }
          frame "K-Line初始化" {
            n161 = global read "Global.vi" "启用K-line诊断"() -> (w186:bool)
            n162 = case shown="真" w186 {
              frame False {
                n163 = local write "STEP"("试验项" ("STEP")) -> ()
              }
              frame True {
                n164 = global read "Global.vi" "VISA resource name"() -> (w192:refnum<visa-resource-name>)
                n165 = global read "Global.vi" "K-Line波特率"() -> (w191:u32)
                n166 = global read "Global.vi" "诊断指令"() -> (w190:string[][])
                n167 = call "K线诊断.vi"("K线诊断"=w190, "波特率"=w191, "VISA resource name"=w192) -> ("字符串"=w188:string, "逻辑与"=w189:bool)  [unwired: 7 in]
                n168 = case shown="假" w189 {
                  tunnel: w188 -> [w197 _]
                  frame False {
                    n169 = global write "Global.vi" "K-Line状态"("NG" ("K-Line状态")) -> ()
                    n170 = call <vilib>:"Three Button Dialog.vi"("Allow user to close window? (TRUE)"=FALSE, "Window Title (\"\")"="K-Line诊断异常" ("Window Title (\"\")"), "Right Button Text (\"Cancel\")"="中止" ("Right Button Text (\"Cancel\")"), "Center Button Text (\"No\")"="忽略" ("Center Button Text (\"No\")"), "Left Button Text (\"Yes\")"="重试" ("Left Button Text (\"Yes\")"), "message"=w197) -> ("Which Button?"=w198:T5)  [unwired: 5 in]
                    n171 = case shown="\"Center Button\"" w198 {
                      frame "Left Button", Default {
                        n172 = local write "STEP"("K-Line初始化" ("STEP")) -> ()
                      }
                      frame "Right Button" {
                        n173 = local write "STEP"("自动退出" ("STEP")) -> ()
                      }
                      frame "Center Button" {
                        n174 = local write "STEP"("试验项" ("STEP")) -> ()
                      }
                    }
                  }
                  frame True {
                    n175 = call "浮动通知.vi"("通知内容"="K-Line诊断正常！") -> ()  [unwired: 11 in]
                    n176 = local write "STEP"("试验项" ("STEP")) -> ()
                    n177 = global write "Global.vi" "K-Line状态"("OK" ("K-Line状态")) -> ()
                  }
                }
              }
            }
          }
          frame "角度标定" {
            n178 = disable-structure shown="启用" {
              disable-tunnel: [w208 "扭矩标定" ("STEP")] -> w207
              frame Disabled {
                n179 = global read "Global.vi" "产品型号"() -> (w209:string)
                n180 = case shown="默认" w209 {
                  tunnel: ["扭矩标定" ("STEP") w211] -> w208
                  frame Default {
                  }
                  frame "R567X" {
                    n181 = while {
                      tunnel: [w212] -> w211
                      stop <- w214 stop-if-true
                      n182 = Wait Until Next ms Multiple(millisecond multiple=u32 100 ("毫秒倍数")) -> ()  [unwired: 1 out]
                      n183 = call "R567X_CAN高级功能.vi"("Function"=T6."角度标定") -> ("完成"=w216:bool)  [unwired: 8 in, 6 out]
                      n184 = case shown="假" w216 {
                        tunnel: [w230 T5."Center Button" ("Which Button?")] -> w215
                        frame False {
                          n185 = global read "Global.vi" "Log"() -> (w224:string)
                          n186 = Concatenate Strings("角度标定失败！\nLOG>>>>>>>" ("message"), "\n", w224) -> (w225:string)
                          n187 = call <vilib>:"Three Button Dialog.vi"("Allow user to close window? (TRUE)"=FALSE, "Right Button Text (\"Cancel\")"="退出" ("Right Button Text (\"Cancel\")"), "Center Button Text (\"No\")"="忽略" ("Center Button Text (\"No\")"), "Left Button Text (\"Yes\")"="重试" ("Left Button Text (\"Yes\")"), "message"=w225) -> ("Which Button?"=w230:T5)  [unwired: 6 in]
                        }
                        frame True {
                        }
                      }
                      n188 = case shown="\"Left Button\", 默认" w215 {
                        tunnel: [FALSE TRUE TRUE] -> w214
                        tunnel: [_ "扭矩标定" ("STEP") "退出自动" ("STEP")] -> w212
                        frame "Left Button", Default {
                        }
                        frame "Center Button" {
                        }
                        frame "Right Button" {
                        }
                      }
                    }
                  }
                }
              }
              frame Enabled {
              }
            }
            n189 = local write "STEP"(w207) -> ()
          }
          frame "角度标定2" {
            n190 = disable-structure shown="启用" {
              disable-tunnel: [w235 "套输入轴花键" ("STEP")] -> w234
              frame Disabled {
                n191 = global read "Global.vi" "产品型号"() -> (w236:string)
                n192 = case shown="默认" w236 {
                  tunnel: ["套输入轴花键" ("STEP") w238] -> w235
                  frame Default {
                  }
                  frame "R567X" {
                    n193 = while {
                      tunnel: [w239] -> w238
                      stop <- w241 stop-if-true
                      n194 = Wait Until Next ms Multiple(millisecond multiple=u32 100 ("毫秒倍数")) -> ()  [unwired: 1 out]
                      n195 = call "R567X_CAN高级功能.vi"("Function"=T6."角度标定") -> ("完成"=w243:bool)  [unwired: 8 in, 6 out]
                      n196 = case shown="假" w243 {
                        tunnel: [w257 T5."Center Button" ("Which Button?")] -> w242
                        frame False {
                          n197 = global read "Global.vi" "Log"() -> (w251:string)
                          n198 = Concatenate Strings("角度标定失败！\nLOG>>>>>>>" ("message"), "\n", w251) -> (w252:string)
                          n199 = call <vilib>:"Three Button Dialog.vi"("Allow user to close window? (TRUE)"=FALSE, "Right Button Text (\"Cancel\")"="退出" ("Right Button Text (\"Cancel\")"), "Center Button Text (\"No\")"="忽略" ("Center Button Text (\"No\")"), "Left Button Text (\"Yes\")"="重试" ("Left Button Text (\"Yes\")"), "message"=w252) -> ("Which Button?"=w257:T5)  [unwired: 6 in]
                        }
                        frame True {
                        }
                      }
                      n200 = case shown="\"Center Button\"" w242 {
                        tunnel: [FALSE TRUE TRUE] -> w241
                        tunnel: [_ "套输入轴花键" ("STEP") "退出自动" ("STEP")] -> w239
                        frame "Left Button", Default {
                        }
                        frame "Center Button" {
                        }
                        frame "Right Button" {
                        }
                      }
                    }
                  }
                }
              }
              frame Enabled {
              }
            }
            n201 = local write "STEP"(w234) -> ()
          }
          frame "扭矩标定" {
            n202 = global read "Global.vi" "产品型号"() -> (w262:string)
            n203 = case shown="\"R567X\"" w262 {
              tunnel: ["试验项" ("STEP") w264] -> w261
              frame Default {
              }
              frame "R567X" {
                n204 = while {
                  tunnel: [w265] -> w264
                  stop <- w267 stop-if-true
                  n205 = Wait Until Next ms Multiple(millisecond multiple=u32 100 ("毫秒倍数")) -> ()  [unwired: 1 out]
                  n206 = call "R567X_CAN高级功能.vi"("Function"=T6."扭矩标定") -> ("完成"=w269:bool)  [unwired: 8 in, 6 out]
                  n207 = case shown="假" w269 {
                    tunnel: [w283 T5."Center Button" ("Which Button?")] -> w268
                    frame False {
                      n208 = global read "Global.vi" "Log"() -> (w277:string)
                      n209 = Concatenate Strings("扭矩标定失败！\nLOG>>>>>>>" ("message"), "\n", w277) -> (w278:string)
                      n210 = call <vilib>:"Three Button Dialog.vi"("Allow user to close window? (TRUE)"=FALSE, "Right Button Text (\"Cancel\")"="退出" ("Right Button Text (\"Cancel\")"), "Center Button Text (\"No\")"="忽略" ("Center Button Text (\"No\")"), "Left Button Text (\"Yes\")"="重试" ("Left Button Text (\"Yes\")"), "message"=w278) -> ("Which Button?"=w283:T5)  [unwired: 6 in]
                    }
                    frame True {
                    }
                  }
                  n211 = case shown="\"Center Button\"" w268 {
                    tunnel: [FALSE TRUE TRUE] -> w267
                    tunnel: [_ "试验项" ("STEP") "退出自动" ("STEP")] -> w265
                    frame "Left Button", Default {
                    }
                    frame "Center Button" {
                    }
                    frame "Right Button" {
                    }
                  }
                }
              }
            }
            n212 = local write "STEP"(w261) -> ()
          }
          frame "试验项" {
            n213 = global read "A180648.vi" "当前检测项"() -> (w286:T4)
            n214 = case shown="默认" w286 {
              selector: w286 -> [w288 _]
              tunnel: [w291 "退输入轴花键" ("STEP")] -> w287
              frame Default {
                n215 = global read "Global.vi" "试验项目"() -> (w289:bool[])
                n216 = Index Array(array=w289, index=w288) -> (element=w290:bool)
                n217 = case shown="真" w290 {
                  tunnel: ["试验项" ("字符串") w298] -> w291
                  tunnel: w288 -> [_ w299]
                  frame False {
                    n218 = global read "A180648.vi" "当前检测项"() -> (w296:T4)
                    n219 = Increment(x=w296) -> (x+1=w295:T4)
                    n220 = global write "A180648.vi" "当前检测项"(w295) -> ()
                    n221 = local read "判定结果"() -> (w292:bool[][])
                    n222 = Build Array (concatenate)(w292, bool[] [FALSE] ("判定结果")) -> (w293:bool[][])
                    n223 = local write "判定结果"(w293) -> ()
                  }
                  frame True {
                    n224 = case shown="\"力特性\"" w299 {
                      tunnel: ["套输入轴花键" ("STEP") "套输入轴花键" ("STEP") "套输入轴花键" ("STEP") "套输入轴花键" ("STEP") w342 "判定" ("STEP") "退输入轴花键" ("STEP") "退输入轴花键" ("STEP")] -> w298
                      frame "空载", Default {
                        n225 = property on="试验项目" class="TabCtl (严格)"("Val(Sgnl)"=T1."空载" ("值(信号)")) -> ()  [unwired: 2 in, 2 out]
                        n226 = call "浮动通知.vi"("通知内容"="空载试验") -> ()  [unwired: 11 in]
                      }
                      frame "功能" {
                        n227 = global write "A180648.vi" "当前车速"(u16 10 ("当前车速")) -> ()
                        n228 = call "浮动通知.vi"("通知内容"="功能试验") -> ()  [unwired: 11 in]
                        n229 = property on="试验项目" class="TabCtl (严格)"("Val(Sgnl)"=T1."功能" ("值(信号)")) -> ()  [unwired: 2 in, 2 out]
                      }
                      frame "力特性" {
                        n230 = global read "A180648.vi" "力特性参数"() -> (w308:sgl[])
                        n231 = call "浮动通知.vi"("通知内容"="力特性试验") -> ()  [unwired: 11 in]
                        n232 = for {
                          tunnel: w308 -> [w311] mode=indexing
                          i -> [w314]
                          w319 = u16 2 items=["byte", "word", "Dword"] ("数据类型")
                          w321 = u8 132 items=["I/O (P)"=128, "Input (I)"=129, "Output (Q)"=130, "Bit Memory (M)"=131, "Data (DB)"=132, "Instance Data (DI)"=133, "Local Data (L)"=134, "Predecessor Local Data (VL)"=135] ("寄存器类型")
                          n233 = Type Cast(type=u32 0 ("写入地址"), x=w311) -> (*(type *) &x=w317:u32)
                          n234 = Multiply(x=w314, y=4) -> (x*y=w315:i32)
                          n235 = Add(x=u32 152 ("写入地址"), y=w315) -> (x+y=w312:u32)
                          n236 = call "Write_Data.vi"("DB #"=u16 7, "寄存器类型"=w321, "写入数据"=w317, "数据类型"=w319, "写入地址"=w312) -> ()  [unwired: 4 in, 3 out]
                        }
                        n237 = property on="试验项目" class="TabCtl (严格)"("Val(Sgnl)"=T1."力特性" ("值(信号)")) -> ()  [unwired: 2 in, 2 out]
                      }
                      frame "传感器特性" {
                        n238 = property on="试验项目" class="TabCtl (严格)"("Val(Sgnl)"=T1."传感器特性" ("值(信号)")) -> ()  [unwired: 2 in, 2 out]
                        n239 = for {
                          tunnel: sgl[] [1.0, 10.0] ("力特性参数") -> [w326] mode=indexing
                          i -> [w329]
                          w334 = u16 2 items=["byte", "word", "Dword"] ("数据类型")
                          w336 = u8 132 items=["I/O (P)"=128, "Input (I)"=129, "Output (Q)"=130, "Bit Memory (M)"=131, "Data (DB)"=132, "Instance Data (DI)"=133, "Local Data (L)"=134, "Predecessor Local Data (VL)"=135] ("寄存器类型")
                          n240 = Type Cast(type=u32 0 ("写入地址"), x=w326) -> (*(type *) &x=w332:u32)
                          n241 = Multiply(x=w329, y=4) -> (x*y=w330:i32)
                          n242 = Add(x=u32 152 ("写入地址"), y=w330) -> (x+y=w327:u32)
                          n243 = call "Write_Data.vi"("DB #"=u16 7, "寄存器类型"=w336, "写入数据"=w332, "数据类型"=w334, "写入地址"=w327) -> ()  [unwired: 4 in, 3 out]
                        }
                        n244 = call "浮动通知.vi"("通知内容"="传感器特性试验") -> ()  [unwired: 11 in]
                      }
                      frame "电流特性" {
                        n245 = global read "Global.vi" "试验项目"() -> (w339:bool[])
                        n246 = call "浮动通知.vi"("通知内容"="电流特性试验") -> ()  [unwired: 11 in]
                        n247 = property on="试验项目" class="TabCtl (严格)"("Val(Sgnl)"=T1."电流特性" ("值(信号)")) -> ()  [unwired: 2 in, 2 out]
                        n248 = Index Array(array=w339, index=2 ("索引")) -> (element=w337:bool)
                        n249 = case shown="假" w337 {
                          tunnel: ["套输入轴花键" ("STEP") "判定" ("STEP")] -> w342
                          frame False {
                          }
                          frame True {
                          }
                        }
                      }
                      frame "振动NVH" {
                        n250 = call "浮动通知.vi"("通知内容"="振动NVH试验") -> ()  [unwired: 11 in]
                        n251 = property on="试验项目" class="TabCtl (严格)"("Val(Sgnl)"=T1."振动NVH" ("值(信号)")) -> ()  [unwired: 2 in, 2 out]
                      }
                      frame "逆向空载" {
                        n252 = global read "A180648.vi" "逆向空载参数"() -> (w349:string[][])
                        n253 = property on="试验项目" class="TabCtl (严格)"("Val(Sgnl)"=T1."逆向空载" ("值(信号)")) -> ()  [unwired: 2 in, 2 out]
                        n254 = call "浮动通知.vi"("通知内容"="逆向空载试验") -> ()  [unwired: 11 in]
                        n255 = Index Array(array=w349, index (col)=1 ("禁用的索引 (列)")) -> (element=w348:string[])  [unwired: 1 in]
                        n256 = for {
                          tunnel: w348 -> [w362] mode=indexing
                          i -> [w356]
                          w364 = u16 2 items=["byte", "word", "Dword"] ("数据类型")
                          w366 = u8 132 items=["I/O (P)"=128, "Input (I)"=129, "Output (Q)"=130, "Bit Memory (M)"=131, "Data (DB)"=132, "Instance Data (DI)"=133, "Local Data (L)"=134, "Predecessor Local Data (VL)"=135] ("寄存器类型")
                          n257 = Fract/Exp String To Number(string=w362, default (0 dbl)=sgl 0.0) -> (number=w360:sgl)  [unwired: 2 in, 1 out]
                          n258 = Multiply(x=w356, y=4) -> (x*y=w357:i32)
                          n259 = Type Cast(type=u32 0 ("写入地址"), x=w360) -> (*(type *) &x=w359:u32)
                          n260 = Add(x=u32 168 ("写入地址"), y=w357) -> (x+y=w354:u32)
                          n261 = call "Write_Data.vi"("DB #"=u16 7, "寄存器类型"=w366, "写入数据"=w359, "数据类型"=w364, "写入地址"=w354) -> ()  [unwired: 4 in, 3 out]
                        }
                      }
                      frame "磨合" {
                        n262 = global read "A180648.vi" "磨合参数"() -> (w369:string[][])
                        n263 = call "浮动通知.vi"("通知内容"="磨合") -> ()  [unwired: 11 in]
                        n264 = property on="试验项目" class="TabCtl (严格)"("Val(Sgnl)"=T1."磨合" ("值(信号)")) -> ()  [unwired: 2 in, 2 out]
                        n265 = Index Array(array=w369, index (col)=1 ("禁用的索引 (列)")) -> (element=w368:string[])  [unwired: 1 in]
                        n266 = for {
                          tunnel: w368 -> [w381] mode=indexing
                          i -> [w375]
                          w383 = u16 2 items=["byte", "word", "Dword"] ("数据类型")
                          w385 = u8 132 items=["I/O (P)"=128, "Input (I)"=129, "Output (Q)"=130, "Bit Memory (M)"=131, "Data (DB)"=132, "Instance Data (DI)"=133, "Local Data (L)"=134, "Predecessor Local Data (VL)"=135] ("寄存器类型")
                          n267 = Fract/Exp String To Number(string=w381, default (0 dbl)=sgl 0.0) -> (number=w379:sgl)  [unwired: 2 in, 1 out]
                          n268 = Multiply(x=w375, y=4) -> (x*y=w376:i32)
                          n269 = Type Cast(type=u32 0 ("写入地址"), x=w379) -> (*(type *) &x=w378:u32)
                          n270 = Add(x=u32 168 ("写入地址"), y=w376) -> (x+y=w373:u32)
                          n271 = call "Write_Data.vi"("DB #"=u16 7, "寄存器类型"=w385, "写入数据"=w378, "数据类型"=w383, "写入地址"=w373) -> ()  [unwired: 4 in, 3 out]
                        }
                      }
                    }
                  }
                }
              }
              frame "完成" {
              }
            }
            n272 = local write "STEP"(w287) -> ()
          }
          frame "判定" {
            n273 = stacked-sequence {
              frame #0 {
                n274 = global read "A180648.vi" "当前检测项"() -> (w387:T4)
                n275 = case shown="\"磨合\"" w387 {
                  frame "完成", Default {
                  }
                  frame "空载" {
                    n276 = global read "判定参数.vi" "空载判定参数"() -> (w399:T9)
                    n277 = local read "空载试验"() -> (w400:cluster{dbl[], dbl[]}[])
                    n278 = global read "Global.vi" "Result"() -> (w398:refnum<vi>)
                    n279 = call "空载试验判定.vi"("Result"=w398, "判定参数"=w399, "XY曲线"=w400) -> ("判定项长度"=w388:i32, "OK？"=w389:bool)  [unwired: 7 in]
                    n280 = global read "A180648.vi" "LED-空载"() -> (w394:refnum<vi>)
                    n281 = local read "判定结果"() -> (w390:bool[][])
                    n282 = Select(t=cluster{u32, u32}[] [{6618880, 6618880}, {6618880, 6618880}, {6618880, 6618880}, {6618880, 6618880}] ("颜色[4]"), s=w389, f=cluster{u32, u32}[] [{16711680, 16711680}, {16711680, 16711680}, {16711680, 16711680}, {16711680, 16711680}] ("颜色[4]")) -> (s? t:f=w395:cluster{u32, u32}[])
                    n283 = Build Array(TRUE, w389) -> (w393:bool[])
                    n284 = global write "判定参数.vi" "空载判定长度"(w388) -> ()
                    n285 = property class="Bool"(reference=w394, "Colors [4]"=w395) -> ()  [unwired: 1 in, 2 out]
                    n286 = Build Array (concatenate)(w390, w393) -> (w391:bool[][])
                    n287 = local write "判定结果"(w391) -> ()
                  }
                  frame "功能" {
                    n288 = local read "功能试验"() -> (w413:cluster{dbl[], dbl[]}[])
                    n289 = global read "判定参数.vi" "功能判定参数"() -> (w412:T10)
                    n290 = global read "Global.vi" "Result"() -> (w411:refnum<vi>)
                    n291 = call "功能试验判定.vi"("Result"=w411, "判定参数"=w412, "XY曲线"=w413) -> ("判定项长度"=w401:i32, "OK？"=w402:bool)  [unwired: 7 in]
                    n292 = global read "A180648.vi" "LED-功能"() -> (w407:refnum<vi>)
                    n293 = local read "判定结果"() -> (w403:bool[][])
                    n294 = Select(t=cluster{u32, u32}[] [{6618880, 6618880}, {6618880, 6618880}, {6618880, 6618880}, {6618880, 6618880}] ("颜色[4]"), s=w402, f=cluster{u32, u32}[] [{16711680, 16711680}, {16711680, 16711680}, {16711680, 16711680}, {16711680, 16711680}] ("颜色[4]")) -> (s? t:f=w408:cluster{u32, u32}[])
                    n295 = global write "判定参数.vi" "功能判定长度"(w401) -> ()
                    n296 = Build Array(TRUE, w402) -> (w406:bool[])
                    n297 = property class="Bool"(reference=w407, "Colors [4]"=w408) -> ()  [unwired: 1 in, 2 out]
                    n298 = Build Array (concatenate)(w403, w406) -> (w404:bool[][])
                    n299 = local write "判定结果"(w404) -> ()
                  }
                  frame "力特性" {
                    n300 = global read "判定参数.vi" "力特性判定参数"() -> (w416:T11)
                    n301 = local read "力特性试验"() -> (w426:cluster{dbl[], dbl[]}[])
                    n302 = for {
                      tunnel: w426 -> [w432]
                      tunnel: [w430] -> w417 mode=indexing
                      tunnel: w416 -> [w429] mode=indexing
                      tunnel: [w427] -> w414 mode=indexing
                      i -> [w428]
                      n303 = global read "Global.vi" "Result"() -> (w431:refnum<vi>)
                      n304 = call "力特性判定.vi"("Result"=w431, "索引"=w428, "判定参数"=w429, "XY曲线"=w432) -> ("判定项长度"=w427:i32, "OK？"=w430:bool)  [unwired: 6 in]
                    }
                    n305 = And Array Elements(Boolean array=w417) -> (logical AND=w415:bool)
                    n306 = global read "A180648.vi" "LED-力特性"() -> (w424:refnum<vi>)
                    n307 = local read "判定结果"() -> (w418:bool[][])
                    n308 = global write "判定参数.vi" "力特性判定长度"(w414) -> ()
                    n309 = Select(t=cluster{u32, u32}[] [{6618880, 6618880}, {6618880, 6618880}, {6618880, 6618880}, {6618880, 6618880}] ("颜色[4]"), s=w415, f=cluster{u32, u32}[] [{16711680, 16711680}, {16711680, 16711680}, {16711680, 16711680}, {16711680, 16711680}] ("颜色[4]")) -> (s? t:f=w425:cluster{u32, u32}[])
                    n310 = Build Array(TRUE, w415) -> (w421:bool[])
                    n311 = property class="Bool"(reference=w424, "Colors [4]"=w425) -> ()  [unwired: 1 in, 2 out]
                    n312 = Build Array (concatenate)(w418, w421) -> (w419:bool[][])
                    n313 = local write "判定结果"(w419) -> ()
                  }
                  frame "传感器特性" {
                    n314 = global read "判定参数.vi" "传感器特性判定参数"() -> (w444:T12)
                    n315 = local read "传感器特性试验"() -> (w445:cluster{dbl[], dbl[]}[])
                    n316 = global read "Global.vi" "Result"() -> (w443:refnum<vi>)
                    n317 = global read "A180648.vi" "LED-传感器特性"() -> (w439:refnum<vi>)
                    n318 = call "传感器特性判定.vi"("Result"=w443, "判定参数"=w444, "XY曲线"=w445) -> ("判定项长度"=w433:i32, "OK？"=w434:bool)  [unwired: 7 in]
                    n319 = local read "判定结果"() -> (w435:bool[][])
                    n320 = Select(t=cluster{u32, u32}[] [{6618880, 6618880}, {6618880, 6618880}, {6618880, 6618880}, {6618880, 6618880}] ("颜色[4]"), s=w434, f=cluster{u32, u32}[] [{16711680, 16711680}, {16711680, 16711680}, {16711680, 16711680}, {16711680, 16711680}] ("颜色[4]")) -> (s? t:f=w440:cluster{u32, u32}[])
                    n321 = Build Array(TRUE, w434) -> (w438:bool[])
                    n322 = global write "判定参数.vi" "传感器特性判定长度"(w433) -> ()
                    n323 = property class="Bool"(reference=w439, "Colors [4]"=w440) -> ()  [unwired: 1 in, 2 out]
                    n324 = Build Array (concatenate)(w435, w438) -> (w436:bool[][])
                    n325 = local write "判定结果"(w436) -> ()
                  }
                  frame "电流特性" {
                    n326 = global read "判定参数.vi" "电流特性判定参数"() -> (w451:T13)
                    n327 = local read "电流特性试验"() -> (w458:cluster{dbl[], dbl[]}[])
                    n328 = for {
                      tunnel: w458 -> [w464]
                      tunnel: [w462] -> w452 mode=indexing
                      tunnel: w451 -> [w461] mode=indexing
                      tunnel: [w459] -> w446 mode=indexing
                      i -> [w460]
                      n329 = global read "Global.vi" "Result"() -> (w463:refnum<vi>)
                      n330 = call "电流特性判定.vi"("Result"=w463, "索引"=w460, "判定参数"=w461, "XY曲线"=w464) -> ("判定项长度"=w459:i32, "OK？"=w462:bool)  [unwired: 6 in]
                    }
                    n331 = And Array Elements(Boolean array=w452) -> (logical AND=w450:bool)
                    n332 = global read "A180648.vi" "LED-电流特性"() -> (w456:refnum<vi>)
                    n333 = local read "判定结果"() -> (w453:bool[][])
                    n334 = Select(t=cluster{u32, u32}[] [{6618880, 6618880}, {6618880, 6618880}, {6618880, 6618880}, {6618880, 6618880}] ("颜色[4]"), s=w450, f=cluster{u32, u32}[] [{16711680, 16711680}, {16711680, 16711680}, {16711680, 16711680}, {16711680, 16711680}] ("颜色[4]")) -> (s? t:f=w457:cluster{u32, u32}[])
                    n335 = global write "判定参数.vi" "电流特性判定长度"(w446) -> ()
                    n336 = Build Array(TRUE, w450) -> (w455:bool[])
                    n337 = property class="Bool"(reference=w456, "Colors [4]"=w457) -> ()  [unwired: 1 in, 2 out]
                    n338 = Build Array (concatenate)(w453, w455) -> (w454:bool[][])
                    n339 = local write "判定结果"(w454) -> ()
                  }
                  frame "振动NVH" {
                    n340 = local read "振动1NVH-FFT"() -> (w467:cluster{"f0":dbl, "df":dbl, "magnitude":dbl[]}[])
                    n341 = local read "振动2NHV-FFT"() -> (w466:cluster{"f0":dbl, "df":dbl, "magnitude":dbl[]}[])
                    n342 = global read "判定参数.vi" "振动判定范围"() -> (w485:T14)
                    n343 = global read "判定参数.vi" "振动判定"() -> (w484:T15)
                    n344 = global read "Global.vi" "Result"() -> (w479:refnum<vi>)
                    n345 = Build Array (concatenate)(w467, w466) -> (w465:cluster{"f0":dbl, "df":dbl, "magnitude":dbl[]}[])
                    n346 = call "振动判定.vi"("Result"=w479, "振动判定"=w484, "振动判定范围"=w485, "FFT"=w465) -> ("判定项长度"=w473:i32, "Limit Specifications"=w471:cluster{"x0":dbl, "dx":dbl, "Y":dbl[]}[][], "FFT 2"=w472:cluster{"f0":dbl, "df":dbl, "magnitude":dbl[]}[], "OK？"=w474:bool)  [unwired: 4 in]
                    n347 = global read "A180648.vi" "LED-振动NVH"() -> (w480:refnum<vi>)
                    n348 = local read "判定结果"() -> (w475:bool[][])
                    n349 = for {
                      tunnel: w472 -> [w488] mode=indexing
                      tunnel: w471 -> [w487] mode=indexing
                      tunnel: [w486] -> w470 mode=indexing
                      n350 = Build Array (concatenate)(w488, w487) -> (w486:cluster{"x0":dbl, "dx":dbl, "Y":dbl[]}[])
                    }
                    n351 = global write "判定参数.vi" "振动判定长度"(w473) -> ()
                    n352 = Select(t=cluster{u32, u32}[] [{6618880, 6618880}, {6618880, 6618880}, {6618880, 6618880}, {6618880, 6618880}] ("颜色[4]"), s=w474, f=cluster{u32, u32}[] [{16711680, 16711680}, {16711680, 16711680}, {16711680, 16711680}, {16711680, 16711680}] ("颜色[4]")) -> (s? t:f=w482:cluster{u32, u32}[])
                    n353 = Build Array(TRUE, w474) -> (w478:bool[])
                    n354 = property class="Bool"(reference=w480, "Colors [4]"=w482) -> ()  [unwired: 1 in, 2 out]
                    n355 = Build Array (concatenate)(w475, w478) -> (w476:bool[][])
                    n356 = local write "判定结果"(w476) -> ()
                    n357 = Index Array(array=w470) -> (element #1=w469:cluster{"x0":dbl, "dx":dbl, "Y":dbl[]}[], element #2=w468:cluster{"x0":dbl, "dx":dbl, "Y":dbl[]}[])  [unwired: 4 in]
                    n358 = local write "振动1NVH-FFT"(w469) -> ()
                    n359 = local write "振动2NHV-FFT"(w468) -> ()
                  }
                  frame "逆向空载" {
                    n360 = global read "判定参数.vi" "逆向空载判定参数"() -> (w500:T16)
                    n361 = local read "逆向空载试验"() -> (w501:cluster{dbl[], dbl[]}[])
                    n362 = global read "Global.vi" "Result"() -> (w499:refnum<vi>)
                    n363 = global read "A180648.vi" "LED-逆向空载"() -> (w495:refnum<vi>)
                    n364 = call "逆向空载试验判定.vi"("Result"=w499, "判定参数"=w500, "XY曲线"=w501) -> ("判定项长度"=w489:i32, "OK？"=w490:bool)  [unwired: 7 in]
                    n365 = Select(t=cluster{u32, u32}[] [{6618880, 6618880}, {6618880, 6618880}, {6618880, 6618880}, {6618880, 6618880}] ("颜色[4]"), s=w490, f=cluster{u32, u32}[] [{16711680, 16711680}, {16711680, 16711680}, {16711680, 16711680}, {16711680, 16711680}] ("颜色[4]")) -> (s? t:f=w496:cluster{u32, u32}[])
                    n366 = property class="Bool"(reference=w495, "Colors [4]"=w496) -> ()  [unwired: 1 in, 2 out]
                    n367 = global write "判定参数.vi" "逆向空载判定长度"(w489) -> ()
                    n368 = local read "判定结果"() -> (w492:bool[][])
                    n369 = Build Array(TRUE, w490) -> (w494:bool[])
                    n370 = Build Array (concatenate)(w492, w494) -> (w493:bool[][])
                    n371 = local write "判定结果"(w493) -> ()
                  }
                  frame "磨合" {
                    w502 = TRUE
                    n372 = global read "A180648.vi" "LED-磨合"() -> (w506:refnum<vi>)
                    n373 = local read "判定结果"() -> (w503:bool[][])
                    n374 = Build Array(w502, w502) -> (w505:bool[])
                    n375 = Build Array (concatenate)(w503, w505) -> (w504:bool[][])
                    n376 = property class="Bool"(reference=w506, "Colors [4]"=cluster{u32, u32}[] [{6618880, 6618880}, {6618880, 6618880}, {6618880, 6618880}, {6618880, 6618880}] ("颜色[4]")) -> ()  [unwired: 1 in, 2 out]
                    n377 = local write "判定结果"(w504) -> ()
                  }
                }
              }
              frame #1 {
                n378 = global read "A180648.vi" "当前检测项"() -> (w509:T4)
                n379 = local write "STEP"("试验项" ("STEP")) -> ()
                n380 = Increment(x=w509) -> (x+1=w510:T4)
                n381 = global write "A180648.vi" "当前检测项"(w510) -> ()
              }
            }
          }
          frame "套输入轴花键" {
            n382 = call "设备状态.vi"() -> ("Status_Read"=w511:i16)  [unwired: 11 in]
            n383 = case shown="1024" w511 {
              frame 0, Default {
                n384 = call "设备状态.vi"("枚举"=enum16{"Read", "Write"}."Write", "Status_Write"=i16 102 ("设备状态")) -> ()  [unwired: 9 in, 1 out]
              }
              frame 103 {
                n385 = global read "A180648.vi" "当前检测项"() -> (w515:T4)
                n386 = case shown="\"力特性\"" w515 {
                  tunnel: ["退输出轴花键" ("STEP") "套输出轴花键" ("STEP") "套输出轴花键" ("STEP") "套输出轴花键" ("STEP") "套输出轴花键" ("STEP")] -> w514
                  frame "空载", Default {
                  }
                  frame "功能" {
                  }
                  frame "力特性" {
                  }
                  frame "传感器特性" {
                  }
                  frame "电流特性" {
                  }
                }
                n387 = local write "STEP"(w514) -> ()
              }
              frame 1024 {
                n388 = local write "STEP"("退出自动" ("STEP")) -> ()
              }
            }
          }
          frame "退输入轴花键" {
            n389 = call "设备状态.vi"() -> ("Status_Read"=w522:i16)  [unwired: 11 in]
            n390 = case shown="105" w522 {
              frame 0, Default {
                n391 = call "设备状态.vi"("枚举"=enum16{"Read", "Write"}."Write", "Status_Write"=i16 104 ("设备状态")) -> ()  [unwired: 9 in, 1 out]
              }
              frame 105 {
                n392 = global read "A180648.vi" "当前检测项"() -> (w526:T4)
                n393 = case shown="\"磨合\"" w526 {
                  tunnel: ["自动" ("STEP") "退输出轴花键" ("STEP") "套输出轴花键" ("STEP") "套输出轴花键" ("STEP") "退输出轴花键" ("STEP")] -> w525
                  frame Default {
                  }
                  frame "振动NVH" {
                  }
                  frame "逆向空载" {
                  }
                  frame "磨合" {
                  }
                  frame "完成" {
                  }
                }
                n394 = local write "STEP"(w525) -> ()
              }
              frame 1024 {
                n395 = local write "STEP"("退出自动" ("STEP")) -> ()
              }
            }
          }
          frame "套输出轴花键" {
            n396 = call "设备状态.vi"() -> ("Status_Read"=w533:i16)  [unwired: 11 in]
            n397 = case shown="107" w533 {
              frame 0, Default {
                n398 = call "设备状态.vi"("枚举"=enum16{"Read", "Write"}."Write", "Status_Write"=i16 106 ("设备状态")) -> ()  [unwired: 9 in, 1 out]
              }
              frame 107 {
                n399 = local write "STEP"("设置输出轴模式" ("STEP")) -> ()
              }
              frame 1024 {
                n400 = local write "STEP"("退出自动" ("STEP")) -> ()
              }
            }
          }
          frame "退输出轴花键" {
            n401 = call "设备状态.vi"() -> ("Status_Read"=w538:i16)  [unwired: 11 in]
            n402 = case shown="109" w538 {
              frame 0, Default {
                n403 = call "设备状态.vi"("枚举"=enum16{"Read", "Write"}."Write", "Status_Write"=i16 108 ("设备状态")) -> ()  [unwired: 9 in, 1 out]
              }
              frame 109 {
                n404 = global read "A180648.vi" "当前检测项"() -> (w541:T4)
                n405 = case shown="\"空载\"" w541 {
                  tunnel: ["自动" ("STEP") "自动" ("STEP") "清除角度标定" ("STEP") "自动" ("STEP")] -> w542
                  frame Default {
                  }
                  frame "振动NVH" {
                    n406 = call "设备状态.vi"("枚举"=enum16{"Read", "Write"}."Write", "Status_Write"=i16 142 ("设备状态")) -> ()  [unwired: 9 in, 1 out]
                  }
                  frame "完成" {
                    n407 = call "设备状态.vi"("枚举"=enum16{"Read", "Write"}."Write", "Status_Write"=i16 160) -> ()  [unwired: 9 in, 1 out]
                    n408 = call "浮动通知.vi"("通知内容"="检测完成！" ("Status")) -> ()  [unwired: 11 in]
                  }
                  frame "空载" {
                    n409 = call "设备状态.vi"("枚举"=enum16{"Read", "Write"}."Write", "Status_Write"=i16 112) -> ()  [unwired: 9 in, 1 out]
                  }
                }
                n410 = local write "STEP"(w542) -> ()
              }
              frame 110 {
                n411 = local write "STEP"("退出自动" ("STEP")) -> ()
              }
            }
          }
          frame "设置输出轴模式" {
            n412 = global read "A180648.vi" "当前检测项"() -> (w556:T4)
            n413 = case shown="\"磨合\"" w556 {
              tunnel: ["自动" ("STEP") "自动" ("STEP") "自动" ("STEP") "自动" ("STEP") "自动" ("STEP") "自动" ("STEP") "自动" ("STEP")] -> w555
              frame Default {
                n414 = disable-structure shown="禁用" {
                  frame Disabled {
                    n415 = call-poly "模式选择.vi"("Max Torque"=200.0, "Velocity"=sgl 0.0) -> ()  [unwired: 9 in, 1 out]
                  }
                  frame Enabled {
                  }
                }
              }
              frame "功能" {
                n416 = stacked-sequence {
                  frame #0 {
                    n417 = call "设备状态.vi"("枚举"=enum16{"Read", "Write"}."Write", "Status_Write"=i16 122 ("设备状态")) -> ()  [unwired: 9 in, 1 out]
                  }
                  frame #1 {
                    n418 = Wait (ms)(milliseconds to wait=u32 500 ("等待时间（毫秒）")) -> ()  [unwired: 1 out]
                  }
                  frame #2 {
                    n419 = global read "A180648.vi" "功能试验参数"() -> (w566:T17)
                    n420 = Unbundle By Name(w566) -> ("负载扭矩"=w564:dbl)
                    n421 = disable-structure shown="禁用" {
                      disable-tunnel: 19.0 ("y") -> [w569 _]
                      disable-tunnel: w564 -> [w568 _]
                      frame Disabled {
                        n422 = Subtract(x=w568, y=w569) -> (x-y=w567:dbl)
                        n423 = call-poly "模式选择.vi"("Max Torque"=w567) -> ()  [unwired: 10 in, 1 out]
                      }
                      frame Enabled {
                      }
                    }
                  }
                }
              }
              frame "力特性" {
                n424 = call "设备状态.vi"("枚举"=enum16{"Read", "Write"}."Write", "Status_Write"=i16 130 ("设备状态")) -> ()  [unwired: 9 in, 1 out]
                n425 = disable-structure shown="禁用" {
                  frame Disabled {
                    n426 = call-poly "模式选择.vi"() -> ()  [unwired: 11 in, 1 out]
                  }
                  frame Enabled {
                  }
                }
              }
              frame "传感器特性" {
                n427 = call "设备状态.vi"("枚举"=enum16{"Read", "Write"}."Write", "Status_Write"=i16 130 ("设备状态")) -> ()  [unwired: 9 in, 1 out]
                n428 = disable-structure shown="禁用" {
                  frame Disabled {
                    n429 = call-poly "模式选择.vi"() -> ()  [unwired: 11 in, 1 out]
                  }
                  frame Enabled {
                  }
                }
              }
              frame "逆向空载" {
                n430 = call "设备状态.vi"("枚举"=enum16{"Read", "Write"}."Write", "Status_Write"=i16 152 ("设备状态")) -> ()  [unwired: 9 in, 1 out]
              }
              frame "磨合" {
                n431 = call "设备状态.vi"("枚举"=enum16{"Read", "Write"}."Write", "Status_Write"=i16 152 ("设备状态")) -> ()  [unwired: 9 in, 1 out]
              }
              frame "电流特性" {
                n432 = call "设备状态.vi"("枚举"=enum16{"Read", "Write"}."Write", "Status_Write"=i16 130 ("设备状态")) -> ()  [unwired: 9 in, 1 out]
              }
            }
            n433 = local write "STEP"(w555) -> ()
          }
          frame "自动" {
            n434 = global read "Global.vi" "设备状态"() -> (w585:i16)
            n435 = case shown="112" w585 {
              frame -128 {
                n436 = disable-structure shown="禁用" {
                  disable-tunnel: [w589 _] -> w586
                  frame Disabled {
                    n437 = call-poly "模式选择.vi"() -> ("error out"=w589:errorcluster)  [unwired: 11 in]
                  }
                  frame Enabled {
                  }
                }
                n438 = global write "Global.vi" "计时开始"(FALSE ("计时开始")) -> ()
                n439 = disable-structure shown="禁用" {
                  disable-tunnel: w586 -> [w590 _]
                  frame Disabled {
                    n440 = call "SetActualPosition.vi"("error in (no error)"=w590) -> ()  [unwired: 10 in, 1 out]
                  }
                  frame Enabled {
                  }
                }
                n441 = call "浮动通知.vi"("通知内容"="复位中……" ("Status")) -> ()  [unwired: 11 in]
              }
              frame Default {
              }
              frame 0 {
                n442 = global write "Global.vi" "计时开始"(FALSE ("计时开始")) -> ()
                n443 = call "浮动通知.vi"("通知内容"="手动状态！" ("Status")) -> ()  [unwired: 11 in]
              }
              frame 1 {
                n444 = call "浮动通知.vi"("通知内容"="请复位！" ("Status")) -> ()  [unwired: 11 in]
              }
              frame 5 {
                n445 = call "浮动通知.vi"("通知内容"="复位完成" ("Status")) -> ()  [unwired: 11 in]
                n446 = global write "Global.vi" "计时开始"(FALSE ("计时开始")) -> ()
              }
              frame 8 {
                n447 = call "浮动通知.vi"("通知内容"="程序停止！" ("Status")) -> ()  [unwired: 11 in]
              }
              frame 100 {
                n448 = call "浮动通知.vi"("通知内容"="请放入产品后按启动夹紧产品！" ("Status")) -> ()  [unwired: 11 in]
              }
              frame 101 {
                n449 = local write "STEP"("扫码" ("STEP")) -> ()
              }
              frame 112 {
                n450 = global read "System_Conf.vi" "system"() -> (w602:T7)
                n451 = call "传感器数据.vi"() -> ("传感器读数"=w609:T18)  [unwired: 10 in, 1 out]
                n452 = local read "空载正向初始化"() -> (w612:bool)
                n453 = Unbundle By Name(w609) -> ("输入编码位移"=w608:sgl, "输入扭矩"=w607:sgl)
                n454 = Unbundle By Name(w602) -> ("空载滤波"=w599:bool, "空载扭矩系数"=w600:dbl)
                n455 = Multiply(x=w600, y=w607) -> (x*y=w601:dbl)
                n456 = case shown="真" w599 {
                  tunnel: w612 -> [_ w620]
                  tunnel: w608 -> [w614 w619]
                  tunnel: w601 -> [w613 w618]
                  tunnel: [w614 w616] -> w606
                  tunnel: [w613 w615] -> w605
                  frame False {
                  }
                  frame True {
                    w617 = 6 ("Averaging Size")
                    n457 = call-poly <userlib>:"MGI Running Average.vi"("Averaging Size"=w617, "Initialize? (F)"=w620, "Value"=w619) -> ("Average"=w616:sgl)  [unwired: 8 in]
                    n458 = call-poly <userlib>:"MGI Running Average.vi"("Averaging Size"=w617, "Initialize? (F)"=w620, "Value"=w618) -> ("Average"=w615:dbl)  [unwired: 8 in]
                  }
                }
                n459 = control-ref of="空载试验"() -> (w611:refnum<vi>)
                n460 = call "曲线采集.vi"("曲线引用"=w611, "曲线索引"=0, "X"=w606, "Y"=w605) -> ("错误输出"=w604:errorcluster)  [unwired: 10 in, 1 out]
                n461 = Unbundle By Name(w604) -> ("status"=w603:bool)
                n462 = local write "空载正向初始化"(w603) -> ()
              }
              frame 113 {
                n463 = local write "STEP"("等待" ("STEP")) -> ()
                n464 = call "设备状态.vi"("枚举"=enum16{"Read", "Write"}."Write", "Status_Write"=i16 114 ("设备状态")) -> ()  [unwired: 9 in, 1 out]
              }
              frame 114 {
                n465 = global read "System_Conf.vi" "system"() -> (w627:T7)
                n466 = call "传感器数据.vi"() -> ("传感器读数"=w634:T18)  [unwired: 10 in, 1 out]
                n467 = Unbundle By Name(w634) -> ("输入编码位移"=w633:sgl, "输入扭矩"=w632:sgl)
                n468 = Unbundle By Name(w627) -> ("空载滤波"=w624:bool, "空载扭矩系数"=w625:dbl)
                n469 = local read "空载逆向初始化"() -> (w637:bool)
                n470 = Multiply(x=w625, y=w632) -> (x*y=w626:dbl)
                n471 = case shown="真" w624 {
                  tunnel: w637 -> [_ w645]
                  tunnel: w633 -> [w639 w644]
                  tunnel: [w639 w642] -> w631
                  tunnel: [w638 w641] -> w630
                  tunnel: w626 -> [w638 w640]
                  frame False {
                  }
                  frame True {
                    w643 = 6 ("Averaging Size")
                    n472 = call-poly <userlib>:"MGI Running Average.vi"("Averaging Size"=w643, "Initialize? (F)"=w645, "Value"=w644) -> ("Average"=w642:sgl)  [unwired: 8 in]
                    n473 = call-poly <userlib>:"MGI Running Average.vi"("Averaging Size"=w643, "Initialize? (F)"=w645, "Value"=w640) -> ("Average"=w641:dbl)  [unwired: 8 in]
                  }
                }
                n474 = control-ref of="空载试验"() -> (w636:refnum<vi>)
                n475 = call "曲线采集.vi"("曲线引用"=w636, "曲线索引"=1, "X"=w631, "Y"=w630) -> ("错误输出"=w629:errorcluster)  [unwired: 10 in, 1 out]
                n476 = Unbundle By Name(w629) -> ("status"=w628:bool)
                n477 = local write "空载逆向初始化"(w628) -> ()
              }
              frame 115 {
                n478 = local write "STEP"("判定" ("STEP")) -> ()
              }
              frame 122 {
                w649 = 4 ("Averaging Size")
                n479 = call "传感器数据.vi"() -> ("传感器读数"=w656:T18)  [unwired: 10 in, 1 out]
                n480 = local read "功能正向初始化"() -> (w648:bool)
                n481 = Unbundle By Name(w656) -> ("输入编码位移"=w654:sgl, "输入扭矩"=w647:sgl, "输出扭矩(大)"=w651:sgl)
                n482 = call-poly <userlib>:"MGI Running Average.vi"("Averaging Size"=w649, "Initialize? (F)"=w648, "Value"=w654) -> ("Average"=w653:sgl)  [unwired: 8 in]
                n483 = call-poly <userlib>:"MGI Running Average.vi"("Averaging Size"=w649, "Initialize? (F)"=w648, "Value"=w647) -> ("Average"=w652:sgl)  [unwired: 8 in]
                n484 = call-poly <userlib>:"MGI Running Average.vi"("Averaging Size"=w649, "Initialize? (F)"=w648, "Value"=w651) -> ("Average"=w650:sgl)  [unwired: 8 in]
                n485 = Greater Or Equal To 0?(x=w653) -> (x >= 0?=w655:bool)
                n486 = case shown="真" w655 {
                  tunnel: w652 -> [_ w674]
                  tunnel: w650 -> [_ w671]
                  tunnel: w653 -> [_ w670]
                  frame False {
                  }
                  frame True {
                    n487 = control-ref of="功能试验"() -> (w673:refnum<vi>)
                    n488 = call "曲线采集.vi"("曲线引用"=w673, "曲线索引"=0, "X"=w670, "Y"=w674) -> ("错误输出"=w669:errorcluster)  [unwired: 10 in, 1 out]
                    n489 = call "曲线采集.vi"("曲线引用"=w673, "曲线索引"=2, "X"=w670, "Y"=w671) -> ()  [unwired: 10 in, 2 out]
                    n490 = Unbundle By Name(w669) -> ("status"=w668:bool)
                    n491 = local write "功能正向初始化"(w668) -> ()
                  }
                }
                n492 = case shown="真" w648 {
                  frame False {
                  }
                  frame True {
                    n493 = control-ref of="振动1NVH-FFT"() -> (w658:refnum<vi>)
                    n494 = control-ref of="振动2NHV-FFT"() -> (w657:refnum<vi>)
                    n495 = vi-ref "NVH_TEST.vi"() -> (w659:refnum<vi>)
                    n496 = property class="VI"(reference=w659) -> (error out=w663:errorcluster, "Name"=w664:string)  [unwired: 1 in, 1 out]
                    n497 = Open VI Reference(type specifier VI Refnum (for type only)=refnum<vi> refnum, vi path=w664, options=128 ("调用并忽略输出"), error in (no error)=w663) -> (vi reference=w661:refnum<vi>)  [unwired: 2 in, 1 out]
                    n498 = call-by-ref "开始异步调用"(reference=w661, "振动NHV-FFT"=w657, "振动NVH-Order"=w658) -> (reference out=w667:refnum<vi>, error out=w665:errorcluster)  [unwired: 11 in]
                    n499 = Close Reference(reference=w667, error in (no error)=w665) -> (error out=w666:errorcluster)
                    n500 = call <vilib>:"Simple Error Handler.vi"("error in (no error)"=w666) -> ()  [unwired: 4 in, 5 out]
                  }
                }
              }
              frame 123 {
                n501 = stacked-sequence {
                  frame #0 {
                    n502 = call "设备状态.vi"("枚举"=enum16{"Read", "Write"}."Write", "Status_Write"=i16 124 ("设备状态")) -> ()  [unwired: 9 in, 1 out]
                  }
                  frame #1 {
                    n503 = global read "A180648.vi" "功能试验参数"() -> (w680:T17)
                    n504 = Unbundle By Name(w680) -> ("负载扭矩"=w679:dbl)
                    n505 = disable-structure shown="禁用" {
                      disable-tunnel: w679 -> [w682 _]
                      disable-tunnel: 19.0 ("y") -> [w681 _]
                      frame Disabled {
                        n506 = Subtract(x=w681, y=w682) -> (x-y=w683:dbl)
                        n507 = call-poly "模式选择.vi"("Max Torque"=w683) -> ()  [unwired: 10 in, 1 out]
                      }
                      frame Enabled {
                      }
                    }
                  }
                }
              }
              frame 124 {
                w690 = 4 ("Averaging Size")
                n508 = call "传感器数据.vi"() -> ("传感器读数"=w697:T18)  [unwired: 10 in, 1 out]
                n509 = local read "功能逆向初始化"() -> (w691:bool)
                n510 = Unbundle By Name(w697) -> ("输入编码位移"=w696:sgl, "输入扭矩"=w684:sgl, "输出扭矩(大)"=w693:sgl)
                n511 = control-ref of="功能试验"() -> (w688:refnum<vi>)
                n512 = call-poly <userlib>:"MGI Running Average.vi"("Averaging Size"=w690, "Initialize? (F)"=w691, "Value"=w684) -> ("Average"=w694:sgl)  [unwired: 8 in]
                n513 = call-poly <userlib>:"MGI Running Average.vi"("Averaging Size"=w690, "Initialize? (F)"=w691, "Value"=w693) -> ("Average"=w692:sgl)  [unwired: 8 in]
                n514 = call-poly <userlib>:"MGI Running Average.vi"("Averaging Size"=w690, "Initialize? (F)"=w691, "Value"=w696) -> ("Average"=w695:sgl)  [unwired: 8 in]
                n515 = call "曲线采集.vi"("曲线引用"=w688, "曲线索引"=1, "X"=w695, "Y"=w694) -> ("错误输出"=w686:errorcluster)  [unwired: 10 in, 1 out]
                n516 = call "曲线采集.vi"("曲线引用"=w688, "曲线索引"=3, "X"=w695, "Y"=w692) -> ()  [unwired: 10 in, 2 out]
                n517 = Unbundle By Name(w686) -> ("status"=w685:bool)
                n518 = local write "功能逆向初始化"(w685) -> ()
              }
              frame 125 {
                n519 = disable-structure shown="禁用" {
                  frame Disabled {
                    n520 = call-poly "模式选择.vi"() -> ()  [unwired: 11 in, 1 out]
                  }
                  frame Enabled {
                  }
                }
                n521 = local write "STEP"("判定" ("STEP")) -> ()
              }
              frame 130 {
                w699 = TRUE
                n522 = global read "A180648.vi" "当前检测项"() -> (w701:T4)
                n523 = case shown="默认" w701 {
                  tunnel: [0 100] -> w700
                  frame Default {
                    w704 = u16 2 items=["byte", "word", "Dword"] ("数据类型")
                    w705 = u8 132 items=["I/O (P)"=128, "Input (I)"=129, "Output (Q)"=130, "Bit Memory (M)"=131, "Data (DB)"=132, "Instance Data (DI)"=133, "Local Data (L)"=134, "Predecessor Local Data (VL)"=135] ("寄存器类型")
                    n524 = global read "A180648.vi" "车速"() -> (w711:sgl[])
                    n525 = Index Array(array=w711) -> (element=w710:sgl)  [unwired: 1 in]
                    n526 = Round Toward +Infinity(x=w710) -> (ceil(x): smallest int >= x=w709:sgl)
                    n527 = Type Cast(type=u32 0, x=w710) -> (*(type *) &x=w712:u32)
                    n528 = To Unsigned Word Integer(number=w709) -> (unsigned 16bit integer=w708:u16)
                    n529 = call "Write_Data.vi"("DB #"=u16 7, "寄存器类型"=w705, "写入数据"=w712, "数据类型"=w704, "写入地址"=u32 160) -> ()  [unwired: 4 in, 3 out]
                    n530 = global write "A180648.vi" "当前车速"(w708) -> ()
                  }
                  frame "传感器特性" {
                    w713 = u32 0
                    w715 = u16 2 items=["byte", "word", "Dword"] ("数据类型")
                    w718 = u8 132 items=["I/O (P)"=128, "Input (I)"=129, "Output (Q)"=130, "Bit Memory (M)"=131, "Data (DB)"=132, "Instance Data (DI)"=133, "Local Data (L)"=134, "Predecessor Local Data (VL)"=135] ("寄存器类型")
                    n531 = global write "A180648.vi" "当前车速"(w713) -> ()
                    n532 = call "Write_Data.vi"("DB #"=u16 7, "寄存器类型"=w718, "写入数据"=w713, "数据类型"=w715, "写入地址"=u32 160) -> ()  [unwired: 4 in, 3 out]
                  }
                }
                n533 = local write "力特性逆向回程"(w699) -> ()
                n534 = local write "力特性正向去程"(w699) -> ()
                n535 = local write "力特性逆向去程"(w699) -> ()
                n536 = local write "力特性正向回程"(w699) -> ()
                n537 = local write "当前车速"(w700) -> ()
              }
              frame 132 {
                n538 = local read "力特性正向去程"() -> (w724:bool)
                n539 = global read "Global.vi" "传感器读数"() -> (w719:T18)
                n540 = control-ref of="传感器特性试验"() -> (w722:refnum<vi>)
                n541 = control-ref of="电流特性试验"() -> (w723:refnum<vi>)
                n542 = local read "当前车速"() -> (w720:i32)
                n543 = control-ref of="力特性试验"() -> (w721:refnum<vi>)
                n544 = case shown="100" w720 {
                  selector: w720 -> [w747 _]
                  tunnel: w719 -> [w752 w768]
                  tunnel: w721 -> [w751 _]
                  tunnel: w722 -> [_ w767]
                  tunnel: w723 -> [w749 _]
                  tunnel: w724 -> [w738 w758]
                  tunnel: [FALSE FALSE] -> w725
                  tunnel: [w739 w762] -> w726
                  tunnel: [w741 _] -> w727
                  tunnel: [w740 _] -> w728
                  tunnel: [_ w761] -> w729
                  tunnel: [_ w760] -> w730
                  tunnel: [_ w759] -> w731
                  tunnel: 20 -> [w737 w757]
                  frame 0, Default {
                    n545 = Unbundle By Name(w752) -> ("输入扭矩"=w750:sgl, "输出扭矩(大)"=w736:sgl, "吸收电流"=w748:sgl)
                    n546 = Multiply(x=w747, y=4) -> (x*y=w744:i32)
                    n547 = call-poly <userlib>:"MGI Running Average.vi"("Averaging Size"=w737, "Initialize? (F)"=w738, "Value"=w748) -> ("Average"=w740:sgl)  [unwired: 8 in]
                    n548 = call-poly <userlib>:"MGI Running Average.vi"("Averaging Size"=w737, "Initialize? (F)"=w738, "Value"=w750) -> ("Average"=w739:sgl)  [unwired: 8 in]
                    n549 = Subtract(x=w736, y=sgl 0.0) -> (x-y=w734:sgl)
                    n550 = Add(x=w744, y=0) -> (x+y=w743:i32)
                    n551 = call-poly <userlib>:"MGI Running Average.vi"("Averaging Size"=w737, "Initialize? (F)"=w738, "Value"=w734) -> ("Average"=w741:sgl)  [unwired: 8 in]
                    n552 = call "曲线采集.vi"("曲线引用"=w749, "曲线索引"=w743, "X"=w739, "Y"=w740) -> ()  [unwired: 10 in, 2 out]
                    n553 = call "曲线采集.vi"("曲线引用"=w751, "曲线索引"=w743, "X"=w739, "Y"=w741) -> ()  [unwired: 10 in, 2 out]
                  }
                  frame 100 {
                    n554 = Unbundle By Name(w768) -> ("输入扭矩"=w754:sgl, "Factorysensor"=w756:sgl, "Factorysensor2"=w755:sgl)
                    n555 = Add(x=w756, y=w755) -> (x+y=w753:sgl)
                    n556 = call-poly <userlib>:"MGI Running Average.vi"("Averaging Size"=w757, "Initialize? (F)"=w758, "Value"=w756) -> ("Average"=w759:sgl)  [unwired: 8 in]
                    n557 = call-poly <userlib>:"MGI Running Average.vi"("Averaging Size"=w757, "Initialize? (F)"=w758, "Value"=w755) -> ("Average"=w760:sgl)  [unwired: 8 in]
                    n558 = call-poly <userlib>:"MGI Running Average.vi"("Averaging Size"=w757, "Initialize? (F)"=w758, "Value"=w754) -> ("Average"=w762:sgl)  [unwired: 8 in]
                    n559 = call-poly <userlib>:"MGI Running Average.vi"("Averaging Size"=w757, "Initialize? (F)"=w758, "Value"=w753) -> ("Average"=w761:sgl)  [unwired: 8 in]
                    n560 = call "曲线采集.vi"("曲线引用"=w767, "曲线索引"=0, "X"=w762, "Y"=w759) -> ()  [unwired: 10 in, 2 out]
                    n561 = call "曲线采集.vi"("曲线引用"=w767, "曲线索引"=1, "X"=w762, "Y"=w760) -> ()  [unwired: 10 in, 2 out]
                    n562 = call "曲线采集.vi"("曲线引用"=w767, "曲线索引"=2, "X"=w762, "Y"=w761) -> ()  [unwired: 10 in, 2 out]
                  }
                }
                n563 = local write "力特性正向去程"(w725) -> ()
                n564 = local write "吸收电流"(w728) -> ()
                n565 = local write "输入扭矩"(w726) -> ()
                n566 = local write "输出扭矩(大)"(w727) -> ()
                n567 = local write "T1+T2"(w729) -> ()
                n568 = local write "T1"(w731) -> ()
                n569 = local write "T2"(w730) -> ()
                "布尔" <- TRUE ("布尔")
              }
              frame 133 {
                n570 = local write "STEP"("等待" ("STEP")) -> ()
                n571 = call "设备状态.vi"("枚举"=enum16{"Read", "Write"}."Write", "Status_Write"=i16 134 ("设备状态")) -> ()  [unwired: 9 in, 1 out]
                n572 = local write "布尔"(TRUE ("布尔")) -> ()
              }
              frame 134 {
                n573 = local read "力特性正向回程"() -> (w778:bool)
                n574 = global read "Global.vi" "传感器读数"() -> (w773:T18)
                n575 = control-ref of="传感器特性试验"() -> (w776:refnum<vi>)
                n576 = control-ref of="电流特性试验"() -> (w777:refnum<vi>)
                n577 = local read "当前车速"() -> (w774:i32)
                n578 = control-ref of="力特性试验"() -> (w775:refnum<vi>)
                n579 = case shown="0, 默认" w774 {
                  selector: w774 -> [w800 _]
                  tunnel: w773 -> [w805 w823]
                  tunnel: w775 -> [w804 _]
                  tunnel: w776 -> [_ w822]
                  tunnel: w777 -> [w802 _]
                  tunnel: w778 -> [w791 w813]
                  tunnel: [FALSE FALSE] -> w779
                  tunnel: [w792 w817] -> w780
                  tunnel: [w794 _] -> w781
                  tunnel: [w793 _] -> w782
                  tunnel: [_ w816] -> w783
                  tunnel: [_ w815] -> w784
                  tunnel: [_ w814] -> w785
                  tunnel: 20 -> [w790 w812]
                  frame 0, Default {
                    n580 = Unbundle By Name(w805) -> ("输入扭矩"=w803:sgl, "输出扭矩(大)"=w789:sgl, "吸收电流"=w801:sgl)
                    n581 = Multiply(x=w800, y=4) -> (x*y=w797:i32)
                    n582 = call-poly <userlib>:"MGI Running Average.vi"("Averaging Size"=w790, "Initialize? (F)"=w791, "Value"=w801) -> ("Average"=w793:sgl)  [unwired: 8 in]
                    n583 = call-poly <userlib>:"MGI Running Average.vi"("Averaging Size"=w790, "Initialize? (F)"=w791, "Value"=w803) -> ("Average"=w792:sgl)  [unwired: 8 in]
                    n584 = Subtract(x=w789, y=sgl 0.0) -> (x-y=w787:sgl)
                    n585 = Add(x=w797, y=1) -> (x+y=w796:i32)
                    n586 = call-poly <userlib>:"MGI Running Average.vi"("Averaging Size"=w790, "Initialize? (F)"=w791, "Value"=w787) -> ("Average"=w794:sgl)  [unwired: 8 in]
                    n587 = call "曲线采集.vi"("曲线引用"=w802, "曲线索引"=w796, "X"=w792, "Y"=w793) -> ()  [unwired: 10 in, 2 out]
                    n588 = call "曲线采集.vi"("曲线引用"=w804, "曲线索引"=w796, "X"=w792, "Y"=w794) -> ()  [unwired: 10 in, 2 out]
                  }
                  frame 100 {
                    n589 = Unbundle By Name(w823) -> ("输入扭矩"=w807:sgl, "Factorysensor"=w810:sgl, "Factorysensor2"=w809:sgl)
                    n590 = Add(x=w810, y=w809) -> (x+y=w811:sgl)
                    n591 = call-poly <userlib>:"MGI Running Average.vi"("Averaging Size"=w812, "Initialize? (F)"=w813, "Value"=w810) -> ("Average"=w814:sgl)  [unwired: 8 in]
                    n592 = call-poly <userlib>:"MGI Running Average.vi"("Averaging Size"=w812, "Initialize? (F)"=w813, "Value"=w809) -> ("Average"=w815:sgl)  [unwired: 8 in]
                    n593 = Multiply(x=1.0, y=w807) -> (x*y=w806:dbl)
                    n594 = call-poly <userlib>:"MGI Running Average.vi"("Averaging Size"=w812, "Initialize? (F)"=w813, "Value"=w806) -> ("Average"=w817:dbl)  [unwired: 8 in]
                    n595 = call-poly <userlib>:"MGI Running Average.vi"("Averaging Size"=w812, "Initialize? (F)"=w813, "Value"=w811) -> ("Average"=w816:sgl)  [unwired: 8 in]
                    n596 = call "曲线采集.vi"("曲线引用"=w822, "曲线索引"=3, "X"=w817, "Y"=w814) -> ()  [unwired: 10 in, 2 out]
                    n597 = call "曲线采集.vi"("曲线引用"=w822, "曲线索引"=4, "X"=w817, "Y"=w815) -> ()  [unwired: 10 in, 2 out]
                    n598 = call "曲线采集.vi"("曲线引用"=w822, "曲线索引"=5, "X"=w817, "Y"=w816) -> ()  [unwired: 10 in, 2 out]
                  }
                }
                n599 = local write "力特性正向回程"(w779) -> ()
                n600 = local write "吸收电流"(w782) -> ()
                n601 = local write "T1"(w785) -> ()
                n602 = local write "输入扭矩"(w780) -> ()
                n603 = local write "T2"(w784) -> ()
                n604 = local write "T1+T2"(w783) -> ()
                n605 = local write "输出扭矩(大)"(w781) -> ()
              }
              frame 135 {
                n606 = local write "STEP"("等待" ("STEP")) -> ()
                n607 = call "设备状态.vi"("枚举"=enum16{"Read", "Write"}."Write", "Status_Write"=i16 136 ("设备状态")) -> ()  [unwired: 9 in, 1 out]
              }
              frame 136 {
                n608 = local read "力特性逆向去程"() -> (w832:bool)
                n609 = global read "Global.vi" "传感器读数"() -> (w827:T18)
                n610 = control-ref of="传感器特性试验"() -> (w830:refnum<vi>)
                n611 = control-ref of="电流特性试验"() -> (w831:refnum<vi>)
                n612 = local read "当前车速"() -> (w828:i32)
                n613 = control-ref of="力特性试验"() -> (w829:refnum<vi>)
                n614 = case shown="0, 默认" w828 {
                  selector: w828 -> [w852 _]
                  tunnel: w827 -> [w857 w875]
                  tunnel: w829 -> [w856 _]
                  tunnel: w830 -> [_ w874]
                  tunnel: w831 -> [w854 _]
                  tunnel: w832 -> [w843 w865]
                  tunnel: [FALSE FALSE] -> w833
                  tunnel: [w844 w869] -> w834
                  tunnel: [w846 _] -> w835
                  tunnel: [w845 _] -> w836
                  tunnel: [_ w868] -> w837
                  tunnel: [_ w867] -> w838
                  tunnel: [_ w866] -> w839
                  tunnel: 10 -> [w842 w864]
                  frame 0, Default {
                    n615 = Unbundle By Name(w857) -> ("输入扭矩"=w855:sgl, "输出扭矩(大)"=w841:sgl, "吸收电流"=w853:sgl)
                    n616 = Multiply(x=w852, y=4) -> (x*y=w849:i32)
                    n617 = call-poly <userlib>:"MGI Running Average.vi"("Averaging Size"=w842, "Initialize? (F)"=w843, "Value"=w853) -> ("Average"=w845:sgl)  [unwired: 8 in]
                    n618 = call-poly <userlib>:"MGI Running Average.vi"("Averaging Size"=w842, "Initialize? (F)"=w843, "Value"=w855) -> ("Average"=w844:sgl)  [unwired: 8 in]
                    n619 = Add(x=w849, y=2) -> (x+y=w848:i32)
                    n620 = call-poly <userlib>:"MGI Running Average.vi"("Averaging Size"=w842, "Initialize? (F)"=w843, "Value"=w841) -> ("Average"=w846:sgl)  [unwired: 8 in]
                    n621 = call "曲线采集.vi"("曲线引用"=w854, "曲线索引"=w848, "X"=w844, "Y"=w845) -> ()  [unwired: 10 in, 2 out]
                    n622 = call "曲线采集.vi"("曲线引用"=w856, "曲线索引"=w848, "X"=w844, "Y"=w846) -> ()  [unwired: 10 in, 2 out]
                  }
                  frame 100 {
                    n623 = Unbundle By Name(w875) -> ("输入扭矩"=w858:sgl, "Factorysensor"=w862:sgl, "Factorysensor2"=w861:sgl)
                    n624 = Add(x=w862, y=w861) -> (x+y=w863:sgl)
                    n625 = call-poly <userlib>:"MGI Running Average.vi"("Averaging Size"=w864, "Initialize? (F)"=w865, "Value"=w862) -> ("Average"=w866:sgl)  [unwired: 8 in]
                    n626 = call-poly <userlib>:"MGI Running Average.vi"("Averaging Size"=w864, "Initialize? (F)"=w865, "Value"=w861) -> ("Average"=w867:sgl)  [unwired: 8 in]
                    n627 = Multiply(x=1.0, y=w858) -> (x*y=w859:dbl)
                    n628 = call-poly <userlib>:"MGI Running Average.vi"("Averaging Size"=w864, "Initialize? (F)"=w865, "Value"=w859) -> ("Average"=w869:dbl)  [unwired: 8 in]
                    n629 = call-poly <userlib>:"MGI Running Average.vi"("Averaging Size"=w864, "Initialize? (F)"=w865, "Value"=w863) -> ("Average"=w868:sgl)  [unwired: 8 in]
                    n630 = call "曲线采集.vi"("曲线引用"=w874, "曲线索引"=6, "X"=w869, "Y"=w866) -> ()  [unwired: 10 in, 2 out]
                    n631 = call "曲线采集.vi"("曲线引用"=w874, "曲线索引"=7, "X"=w869, "Y"=w867) -> ()  [unwired: 10 in, 2 out]
                    n632 = call "曲线采集.vi"("曲线引用"=w874, "曲线索引"=8, "X"=w869, "Y"=w868) -> ()  [unwired: 10 in, 2 out]
                  }
                }
                n633 = local write "力特性逆向去程"(w833) -> ()
                n634 = local write "吸收电流"(w836) -> ()
                n635 = local write "T1"(w839) -> ()
                n636 = local write "输入扭矩"(w834) -> ()
                n637 = local write "T2"(w838) -> ()
                n638 = local write "T1+T2"(w837) -> ()
                n639 = local write "输出扭矩(大)"(w835) -> ()
              }
              frame 137 {
                n640 = call "设备状态.vi"("枚举"=enum16{"Read", "Write"}."Write", "Status_Write"=i16 138 ("设备状态")) -> ()  [unwired: 9 in, 1 out]
                n641 = local write "STEP"("等待" ("STEP")) -> ()
              }
              frame 138 {
                n642 = control-ref of="电流特性试验"() -> (w884:refnum<vi>)
                n643 = local read "当前车速"() -> (w881:i32)
                n644 = global read "Global.vi" "传感器读数"() -> (w880:T18)
                n645 = control-ref of="力特性试验"() -> (w882:refnum<vi>)
                n646 = control-ref of="传感器特性试验"() -> (w883:refnum<vi>)
                n647 = local read "力特性逆向回程"() -> (w885:bool)
                n648 = case shown="100" w881 {
                  selector: w881 -> [w906 _]
                  tunnel: w880 -> [w911 w929]
                  tunnel: w882 -> [w910 _]
                  tunnel: w883 -> [_ w928]
                  tunnel: w884 -> [w908 _]
                  tunnel: w885 -> [w897 w919]
                  tunnel: [FALSE FALSE] -> w886
                  tunnel: [w898 w923] -> w887
                  tunnel: [w900 _] -> w888
                  tunnel: [w899 _] -> w889
                  tunnel: [_ w922] -> w890
                  tunnel: [_ w921] -> w891
                  tunnel: [_ w920] -> w892
                  tunnel: 10 -> [w896 w918]
                  frame 0, Default {
                    n649 = Unbundle By Name(w911) -> ("输入扭矩"=w909:sgl, "输出扭矩(大)"=w895:sgl, "吸收电流"=w907:sgl)
                    n650 = Multiply(x=w906, y=4) -> (x*y=w903:i32)
                    n651 = Subtract(x=w895, y=sgl 0.0) -> (x-y=w893:sgl)
                    n652 = call-poly <userlib>:"MGI Running Average.vi"("Averaging Size"=w896, "Initialize? (F)"=w897, "Value"=w907) -> ("Average"=w899:sgl)  [unwired: 8 in]
                    n653 = call-poly <userlib>:"MGI Running Average.vi"("Averaging Size"=w896, "Initialize? (F)"=w897, "Value"=w893) -> ("Average"=w900:sgl)  [unwired: 8 in]
                    n654 = call-poly <userlib>:"MGI Running Average.vi"("Averaging Size"=w896, "Initialize? (F)"=w897, "Value"=w909) -> ("Average"=w898:sgl)  [unwired: 8 in]
                    n655 = Add(x=w903, y=3) -> (x+y=w902:i32)
                    n656 = call "曲线采集.vi"("曲线引用"=w908, "曲线索引"=w902, "X"=w898, "Y"=w899) -> ()  [unwired: 10 in, 2 out]
                    n657 = call "曲线采集.vi"("曲线引用"=w910, "曲线索引"=w902, "X"=w898, "Y"=w900) -> ()  [unwired: 10 in, 2 out]
                  }
                  frame 100 {
                    n658 = Unbundle By Name(w929) -> ("输入扭矩"=w913:sgl, "Factorysensor"=w916:sgl, "Factorysensor2"=w915:sgl)
                    n659 = Multiply(x=1.0, y=w913) -> (x*y=w912:dbl)
                    n660 = Add(x=w916, y=w915) -> (x+y=w917:sgl)
                    n661 = call-poly <userlib>:"MGI Running Average.vi"("Averaging Size"=w918, "Initialize? (F)"=w919, "Value"=w912) -> ("Average"=w923:dbl)  [unwired: 8 in]
                    n662 = call-poly <userlib>:"MGI Running Average.vi"("Averaging Size"=w918, "Initialize? (F)"=w919, "Value"=w917) -> ("Average"=w922:sgl)  [unwired: 8 in]
                    n663 = call-poly <userlib>:"MGI Running Average.vi"("Averaging Size"=w918, "Initialize? (F)"=w919, "Value"=w916) -> ("Average"=w920:sgl)  [unwired: 8 in]
                    n664 = call-poly <userlib>:"MGI Running Average.vi"("Averaging Size"=w918, "Initialize? (F)"=w919, "Value"=w915) -> ("Average"=w921:sgl)  [unwired: 8 in]
                    n665 = call "曲线采集.vi"("曲线引用"=w928, "曲线索引"=11, "X"=w923, "Y"=w922) -> ()  [unwired: 10 in, 2 out]
                    n666 = call "曲线采集.vi"("曲线引用"=w928, "曲线索引"=9, "X"=w923, "Y"=w920) -> ()  [unwired: 10 in, 2 out]
                    n667 = call "曲线采集.vi"("曲线引用"=w928, "曲线索引"=10, "X"=w923, "Y"=w921) -> ()  [unwired: 10 in, 2 out]
                  }
                }
                n668 = local write "力特性逆向回程"(w886) -> ()
                n669 = local write "吸收电流"(w889) -> ()
                n670 = local write "输入扭矩"(w887) -> ()
                n671 = local write "输出扭矩(大)"(w888) -> ()
                n672 = local write "T1+T2"(w890) -> ()
                n673 = local write "T1"(w892) -> ()
                n674 = local write "T2"(w891) -> ()
              }
              frame 139 {
                n675 = local read "布尔"() -> (w930:bool)
                n676 = global write "A180648.vi" "布尔"(w930) -> ()
                n677 = case shown="真" w930 {
                  frame False {
                  }
                  frame True {
                    n678 = global read "A180648.vi" "车速"() -> (w935:sgl[])
                    n679 = local write "布尔"(FALSE ("布尔")) -> ()
                    n680 = Array Size(array=w935) -> (size(s)=w936:i32)
                    n681 = local read "当前车速"() -> (w931:i32)
                    n682 = Decrement(x=w936) -> (x-1=w934:i32)
                    n683 = Greater Or Equal?(x=w931, y=w934) -> (x >= y?=w932:bool)
                    n684 = global write "A180648.vi" "139select"(w932) -> ()
                    n685 = case shown="假" w932 {
                      frame False {
                        n686 = stacked-sequence {
                          frame #0 {
                            n687 = local read "当前车速"() -> (w938:i32)
                            n688 = Increment(x=w938) -> (x+1=w937:i32)
                            n689 = local write "当前车速"(w937) -> ()
                          }
                          frame #1 {
                            w946 = u16 2 items=["byte", "word", "Dword"] ("数据类型")
                            w949 = u8 132 items=["I/O (P)"=128, "Input (I)"=129, "Output (Q)"=130, "Bit Memory (M)"=131, "Data (DB)"=132, "Instance Data (DI)"=133, "Local Data (L)"=134, "Predecessor Local Data (VL)"=135] ("寄存器类型")
                            n690 = global read "A180648.vi" "车速"() -> (w943:sgl[])
                            n691 = local read "当前车速"() -> (w942:i32)
                            n692 = Index Array(array=w943, index=w942) -> (element=w939:sgl)
                            n693 = Type Cast(type=u32 0, x=w939) -> (*(type *) &x=w944:u32)
                            n694 = Round Toward +Infinity(x=w939) -> (ceil(x): smallest int >= x=w941:sgl)
                            n695 = call "Write_Data.vi"("DB #"=u16 7, "寄存器类型"=w949, "写入数据"=w944, "数据类型"=w946, "写入地址"=u32 160) -> ()  [unwired: 4 in, 3 out]
                            n696 = To Unsigned Word Integer(number=w941) -> (unsigned 16bit integer=w940:u16)
                            n697 = global write "A180648.vi" "当前车速"(w940) -> ()
                          }
                          frame #2 {
                            n698 = call "设备状态.vi"("枚举"=enum16{"Read", "Write"}."Write", "Status_Write"=i16 132 ("设备状态")) -> ()  [unwired: 9 in, 1 out]
                          }
                          frame #3 {
                            w952 = TRUE
                            n699 = local write "力特性逆向回程"(w952) -> ()
                            n700 = local write "力特性正向去程"(w952) -> ()
                            n701 = local write "力特性逆向去程"(w952) -> ()
                            n702 = local write "力特性正向回程"(w952) -> ()
                          }
                        }
                      }
                      frame True {
                        n703 = local write "STEP"("判定" ("STEP")) -> ()
                      }
                    }
                    n704 = global write "A180648.vi" "v"(w931) -> ()
                  }
                }
              }
              frame 142 {
                n705 = stacked-sequence {
                  frame #0 {
                    n706 = disable-structure shown="禁用" {
                      frame Disabled {
                        n707 = global read "Global.vi" "输出占空比"() -> (w957:refnum<vi>)
                        n708 = property class="Num"(reference=w957, "Val(Sgnl)"=52.0) -> ()  [unwired: 1 in, 2 out]
                      }
                      frame Enabled {
                      }
                    }
                    n709 = call "设备状态.vi"("枚举"=enum16{"Read", "Write"}."Write", "Status_Write"=i16 143) -> ()  [unwired: 9 in, 1 out]
                  }
                  frame #1 {
                    n710 = Wait (ms)(milliseconds to wait=u32 2000 ("等待时间（毫秒）")) -> ()  [unwired: 1 out]
                  }
                }
              }
              frame 143 {
                n711 = stacked-sequence {
                  frame #0 {
                    n712 = call "DaqClose.vi"() -> ()  [unwired: 11 in, 1 out]
                  }
                  frame #1 {
                    n713 = control-ref of="振动1NVH-FFT"() -> (w960:refnum<vi>)
                    n714 = control-ref of="振动2NHV-FFT"() -> (w959:refnum<vi>)
                    n715 = call "振动检测.vi"("振动一"=w960, "通道输入"=tag "cDAQ1Mod1/ai1:2" ("DAQmx物理通道"), "振动二"=w959, "重置"=FALSE) -> ("spectrum info"=w963:T19[])  [unwired: 10 in, 1 out]
                    n716 = global write "Global.vi" "spectrum info"(w963) -> ()
                  }
                  frame #2 {
                    n717 = Wait (ms)(milliseconds to wait=u32 2000 ("等待时间（毫秒）")) -> ()  [unwired: 1 out]
                  }
                  frame #3 {
                    n718 = disable-structure shown="禁用" {
                      frame Disabled {
                        n719 = global read "Global.vi" "输出占空比"() -> (w968:refnum<vi>)
                        n720 = property class="Num"(reference=w968, "Val(Sgnl)"=48.0) -> ()  [unwired: 1 in, 2 out]
                      }
                      frame Enabled {
                      }
                    }
                    n721 = call "设备状态.vi"("枚举"=enum16{"Read", "Write"}."Write", "Status_Write"=i16 145) -> ()  [unwired: 9 in, 1 out]
                    n722 = call "DaqClose.vi"() -> ()  [unwired: 11 in, 1 out]
                  }
                  frame #4 {
                    n723 = Wait (ms)(milliseconds to wait=u32 2000 ("等待时间（毫秒）")) -> ()  [unwired: 1 out]
                  }
                }
              }
              frame 144 {
                n724 = stacked-sequence {
                  frame #0 {
                    n725 = control-ref of="振动1NVH-FFT"() -> (w971:refnum<vi>)
                    n726 = control-ref of="振动2NHV-FFT"() -> (w970:refnum<vi>)
                    n727 = call "振动检测.vi"("振动一"=w971, "通道输入"=tag "cDaq1Mod1/ai1:2" ("DAQmx物理通道"), "振动二"=w970, "重置"=FALSE) -> ("spectrum info"=w974:T19[])  [unwired: 10 in, 1 out]
                    n728 = global write "Global.vi" "spectrum info"(w974) -> ()
                  }
                  frame #1 {
                    n729 = call "设备状态.vi"("枚举"=enum16{"Read", "Write"}."Write", "Status_Write"=i16 145) -> ()  [unwired: 9 in, 1 out]
                  }
                }
              }
              frame 146 {
                n730 = local write "STEP"("判定" ("STEP")) -> ()
              }
              frame 152 {
                n731 = global read "A180648.vi" "当前检测项"() -> (w978:T4)
                n732 = case shown="\"逆向空载\", 默认" w978 {
                  frame "逆向空载", Default {
                    n733 = global read "System_Conf.vi" "system"() -> (w988:T7)
                    n734 = call "传感器数据.vi"() -> ("传感器读数"=w979:T18)  [unwired: 10 in, 1 out]
                    n735 = Unbundle By Name(w988) -> ("逆向空载滤波"=w991:bool, "逆向空载扭矩系数"=w990:dbl)
                    n736 = Unbundle By Name(w979) -> ("输出轴旋转角度"=w986:sgl, "输出扭矩(小)"=w987:sgl)
                    n737 = local read "逆向空载正向初始化"() -> (w981:bool)
                    n738 = Multiply(x=w987, y=w990) -> (x*y=w989:dbl)
                    n739 = case shown="真" w991 {
                      tunnel: [w993 w1000] -> w980
                      tunnel: w981 -> [_ w999]
                      tunnel: [w994 w997] -> w985
                      tunnel: w986 -> [w994 w996]
                      tunnel: w989 -> [w993 w995]
                      frame False {
                      }
                      frame True {
                        w998 = 10 ("Averaging Size")
                        n740 = call-poly <userlib>:"MGI Running Average.vi"("Averaging Size"=w998, "Initialize? (F)"=w999, "Value"=w996) -> ("Average"=w997:sgl)  [unwired: 8 in]
                        n741 = call-poly <userlib>:"MGI Running Average.vi"("Averaging Size"=w998, "Initialize? (F)"=w999, "Value"=w995) -> ("Average"=w1000:dbl)  [unwired: 8 in]
                      }
                    }
                    n742 = control-ref of="逆向空载试验"() -> (w992:refnum<vi>)
                    n743 = call "曲线采集.vi"("曲线引用"=w992, "曲线索引"=0, "X"=w985, "Y"=w980) -> ("错误输出"=w983:errorcluster)  [unwired: 10 in, 1 out]
                    n744 = Unbundle By Name(w983) -> ("status"=w984:bool)
                    n745 = local write "逆向空载正向初始化"(w984) -> ()
                  }
                  frame "磨合" {
                    w1001 = 10 ("Averaging Size")
                    n746 = call "传感器数据.vi"() -> ("传感器读数"=w1004:T18)  [unwired: 10 in, 1 out]
                    n747 = Unbundle By Name(w1004) -> ("输出轴旋转角度"=w1010:sgl, "输出扭矩(大)"=w1011:sgl)
                    n748 = local read "磨合正向初始化"() -> (w1006:bool)
                    n749 = control-ref of="磨合"() -> (w1002:refnum<vi>)
                    n750 = call-poly <userlib>:"MGI Running Average.vi"("Averaging Size"=w1001, "Initialize? (F)"=w1006, "Value"=w1010) -> ("Average"=w1009:sgl)  [unwired: 8 in]
                    n751 = call-poly <userlib>:"MGI Running Average.vi"("Averaging Size"=w1001, "Initialize? (F)"=w1006, "Value"=w1011) -> ("Average"=w1005:sgl)  [unwired: 8 in]
                    n752 = call "曲线采集.vi"("曲线引用"=w1002, "曲线索引"=0, "X"=w1009, "Y"=w1005) -> ("错误输出"=w1007:errorcluster)  [unwired: 10 in, 1 out]
                    n753 = Unbundle By Name(w1007) -> ("status"=w1008:bool)
                    n754 = local write "磨合正向初始化"(w1008) -> ()
                  }
                }
              }
              frame 153 {
                n755 = call "设备状态.vi"("枚举"=enum16{"Read", "Write"}."Write", "Status_Write"=i16 154) -> ()  [unwired: 9 in, 1 out]
              }
              frame 154 {
                n756 = global read "A180648.vi" "当前检测项"() -> (w1014:T4)
                n757 = case shown="\"逆向空载\", 默认" w1014 {
                  frame "逆向空载", Default {
                    n758 = global read "System_Conf.vi" "system"() -> (w1026:T7)
                    n759 = call "传感器数据.vi"() -> ("传感器读数"=w1019:T18)  [unwired: 10 in, 1 out]
                    n760 = Unbundle By Name(w1026) -> ("逆向空载滤波"=w1028:bool, "逆向空载扭矩系数"=w1027:dbl)
                    n761 = Unbundle By Name(w1019) -> ("输出轴旋转角度"=w1021:sgl, "输出扭矩(小)"=w1024:sgl)
                    n762 = local read "逆向空载逆向初始化"() -> (w1020:bool)
                    n763 = Multiply(x=w1024, y=w1027) -> (x*y=w1025:dbl)
                    n764 = case shown="真" w1028 {
                      tunnel: w1020 -> [_ w1036]
                      tunnel: w1021 -> [w1030 w1035]
                      tunnel: [w1030 w1034] -> w1022
                      tunnel: [w1029 w1033] -> w1023
                      tunnel: w1025 -> [w1029 w1031]
                      frame False {
                      }
                      frame True {
                        w1032 = 10 ("Averaging Size")
                        n765 = call-poly <userlib>:"MGI Running Average.vi"("Averaging Size"=w1032, "Initialize? (F)"=w1036, "Value"=w1035) -> ("Average"=w1034:sgl)  [unwired: 8 in]
                        n766 = call-poly <userlib>:"MGI Running Average.vi"("Averaging Size"=w1032, "Initialize? (F)"=w1036, "Value"=w1031) -> ("Average"=w1033:dbl)  [unwired: 8 in]
                      }
                    }
                    n767 = control-ref of="逆向空载试验"() -> (w1015:refnum<vi>)
                    n768 = call "曲线采集.vi"("曲线引用"=w1015, "曲线索引"=1, "X"=w1022, "Y"=w1023) -> ("错误输出"=w1017:errorcluster)  [unwired: 10 in, 1 out]
                    n769 = Unbundle By Name(w1017) -> ("status"=w1018:bool)
                    n770 = local write "逆向空载逆向初始化"(w1018) -> ()
                  }
                  frame "磨合" {
                    w1037 = 10 ("Averaging Size")
                    n771 = call "传感器数据.vi"() -> ("传感器读数"=w1041:T18)  [unwired: 10 in, 1 out]
                    n772 = Unbundle By Name(w1041) -> ("输出轴旋转角度"=w1043:sgl, "输出扭矩(大)"=w1046:sgl)
                    n773 = local read "磨合逆向初始化"() -> (w1042:bool)
                    n774 = control-ref of="磨合"() -> (w1047:refnum<vi>)
                    n775 = call-poly <userlib>:"MGI Running Average.vi"("Averaging Size"=w1037, "Initialize? (F)"=w1042, "Value"=w1043) -> ("Average"=w1044:sgl)  [unwired: 8 in]
                    n776 = call-poly <userlib>:"MGI Running Average.vi"("Averaging Size"=w1037, "Initialize? (F)"=w1042, "Value"=w1046) -> ("Average"=w1045:sgl)  [unwired: 8 in]
                    n777 = call "曲线采集.vi"("曲线引用"=w1047, "曲线索引"=1, "X"=w1044, "Y"=w1045) -> ("错误输出"=w1039:errorcluster)  [unwired: 10 in, 1 out]
                    n778 = Unbundle By Name(w1039) -> ("status"=w1040:bool)
                    n779 = local write "磨合逆向初始化"(w1040) -> ()
                  }
                }
              }
              frame 155 {
                n780 = local write "STEP"("判定" ("STEP")) -> ()
              }
              frame 999 {
                n781 = call "浮动通知.vi"("通知内容"="请启动！" ("Status")) -> ()  [unwired: 11 in]
              }
              frame 1000 {
                n782 = local write "STEP"("初始化" ("STEP")) -> ()
              }
              frame 1024 {
                n783 = local write "STEP"("退出自动" ("STEP")) -> ()
              }
            }
          }
          frame "合格判定" {
            n784 = Wait (ms)(milliseconds to wait=u32 100 ("等待时间（毫秒）")) -> ()  [unwired: 1 out]
            n785 = local write "STEP"("等待" ("STEP")) -> ()
          }
          frame "清除角度标定" {
            n786 = disable-structure shown="禁用" {
              frame Disabled {
                n787 = global read "Global.vi" "产品型号"() -> (w1055:string)
                n788 = case shown="\"R567X\"" w1055 {
                  tunnel: ["报表" ("STEP") w1057] -> w1054
                  frame Default {
                  }
                  frame "R567X" {
                    n789 = while {
                      tunnel: [w1058] -> w1057
                      stop <- w1060 stop-if-true
                      n790 = Wait Until Next ms Multiple(millisecond multiple=u32 100 ("毫秒倍数")) -> ()  [unwired: 1 out]
                      n791 = call "R567X_CAN高级功能.vi"("Function"=T6."角度标定清除") -> ("完成"=w1062:bool)  [unwired: 8 in, 6 out]
                      n792 = case shown="真" w1062 {
                        tunnel: [w1070 FALSE ("T button?")] -> w1061
                        frame False {
                          n793 = Two Button Dialog(message="角度标定清除失败！\n是否重试？", 1:"忽略" ("Center Button Text (\"No\")"), 2:"重试" ("Left Button Text (\"Yes\")")) -> (T button?=w1070:bool)
                        }
                        frame True {
                        }
                      }
                      n794 = case shown="假" w1061 {
                        tunnel: [FALSE TRUE] -> w1060
                        tunnel: [_ "报表" ("STEP")] -> w1058
                        frame True {
                        }
                        frame False {
                        }
                      }
                    }
                  }
                }
                n795 = local write "STEP"(w1054) -> ()
              }
              frame Enabled {
                n796 = local write "STEP"("报表" ("STEP")) -> ()
              }
            }
          }
          frame "报表" {
            n797 = stacked-sequence {
              frame #0 {
                n798 = global write "Global.vi" "计时开始"(FALSE ("计时开始")) -> ()
                n799 = global write "Global.vi" "CAN_STOP"(TRUE ("CAN_STOP")) -> ()
                n800 = vi-ref "CAN.vi"() -> (w1076:refnum<vi>)
                n801 = invoke class="VI" method="Ctrl Val.Set"(reference=w1076, "Control Name"="Stop" ("控件名"), "Value"=TRUE) -> ()  [unwired: 2 in, 5 out]
              }
              frame #1 {
                n802 = call <vilib>:"Space Constant.vi"() -> ("String"=w1080:string)
                n803 = global read "Global.vi" "产品编号"() -> (w1079:string)
                n804 = call "时间秒.vi"() -> ("结果字符串"=w1081:string)  [unwired: 11 in]
                n805 = Concatenate Strings(w1079, w1080, w1081) -> (w1078:string)
                n806 = call "Report.vi"("文件重命名"=TRUE, "文件名称"=w1078, "检测结果"="判定结果") -> ("error out"=w1085:errorcluster, "PRODUCT_VAULE"=w1083:string)  [unwired: 7 in]
                n807 = global read "Global.vi" "联机模式"() -> (w1087:enum16{"单机", "追溯"})
                n808 = call <vilib>:"Simple Error Handler.vi"("error in (no error)"=w1085) -> ("error out"=w1082:errorcluster)  [unwired: 4 in, 4 out]
                n809 = case shown="\"追溯\"" w1087 {
                  tunnel: w1083 -> [_ w1089]
                  tunnel: w1082 -> [_ w1088]
                  frame "单机", Default {
                  }
                  frame "追溯" {
                    n810 = global read "追溯Global.vi" "DEVICE_ID"() -> (w1098:string)
                    n811 = global read "追溯Global.vi" "CODE_ID"() -> (w1099:string)
                    n812 = global read "追溯Global.vi" "USER_ID"() -> (w1097:string)
                    n813 = global read "Global.vi" "Result"() -> (w1091:refnum<vi>)
                    n814 = call "UPRESULT.vi"("DEVICE_ID"=w1098, "USER_ID"=w1097, "CODE_ID"=w1099, "RESULT_VALUE"=w1089, "错误输入"=w1088) -> ()  [unwired: 10 in, 1 out]
                    n815 = property class="Tbl"(reference=w1091) -> (reference out=w1096:refnum<vi>, error out=w1093:errorcluster, "Row Headers[]"=w1094:string[])  [unwired: 1 in]
                    n816 = property class="Tbl"(reference=w1096, error in=w1093) -> (error out=w1092:errorcluster, "Value"=w1095:string[][])  [unwired: 1 out]
                    n817 = for {
                      tunnel: w1095 -> [w1103] mode=indexing
                      tunnel: w1094 -> [w1104] mode=indexing
                      tunnel: [w1101] -> w1090 mode=indexing if=w1102
                      shift-right: [w1100] -> _
                      shift-left: w1092 -> [w1100]
                      n818 = Build Array (concatenate)(w1104, w1103) -> (w1101:string[])
                      n819 = Index Array(array=w1103) -> (element=w1105:string)  [unwired: 1 in]
                      n820 = case shown="\"\"" w1105 {
                        tunnel: [TRUE FALSE] -> w1102
                        frame Default {
                        }
                        frame "" {
                        }
                      }
                    }
                    n821 = call "UPTEST.vi"("Result"=w1090, "CODE_ID"=w1099, "DEVICE_ID"=w1098) -> ()  [unwired: 6 in, 1 out]
                  }
                }
              }
              frame #2 {
                n822 = local write "STEP"("进入自动" ("STEP")) -> ()
              }
            }
          }
        }
        n823 = global read "Global.vi" "程序关闭"() -> (w36:bool)
      }
      n824 = while {
        shift-right: [w1109] -> w33
        shift-left: w34 -> [w1110]
        stop <- w1111 stop-if-true
        n825 = event shown="[6] \"电流特性试验\", \"传感器特性试验\", \"力特性试验\", \"空载试验\", \"功能试验\", \"逆向空载试验\", \"磨合\": 鼠标进入;  \"电流特性试验\", \"传感器特性试验\", \"力特性试验\", \"空载试验\", \"功能试验\", \"逆向空载试验\", \"磨合\": 鼠标离开;  \"电流特性试验\", \"传感器特性试验\", \"力特性试验\", \"空载试验\", \"功能试验\", \"逆向空载试验\": 游标移动;  \"磨合\": 鼠标移动" {
          selector: w1110 -> [_ _ _ _ _ _ _ _]
          dyn-events: [_ _ _ _ _ _ _ _] -> w1109
          timeout: 200 -> [_ _ _ _ _ _ _ _]
          event Timeout {
            n826 = event-data() -> ()  [unwired: 1 in, 3 out]
            n827 = disable-structure shown="禁用" {
              frame Disabled {
                n828 = call "Obtain Broadcast Events for Registration.vi"() -> ("Already running?"=w1113:bool)  [unwired: 9 in, 2 out]
                n829 = case shown="真" w1113 {
                  frame False {
                    n830 = local write "STEP"("手动" ("STEP")) -> ()
                  }
                  frame True {
                    n831 = call "错误代码.vi"() -> ("Status_Read"=w1115:u32)  [unwired: 11 in]
                    n832 = feedback #1() -> (w1125:u32)  [unwired: 1 in]
                    n833 = feedback-in #1(w1115) -> ()
                    n834 = case shown="1, 默认" w1115 {
                      frame 0 {
                        n835 = global read "Global.vi" "报警图标"() -> (w1126:refnum<vi>)
                        n836 = property class="Bool"(reference=w1126, "Visible"=FALSE ("可见")) -> ()  [unwired: 1 in, 2 out]
                      }
                      frame 1, Default {
                        n837 = global read "Global.vi" "报警图标"() -> (w1129:refnum<vi>)
                        n838 = property class="Bool"(reference=w1129, "Visible"=TRUE ("可见")) -> ()  [unwired: 1 in, 2 out]
                      }
                    }
                    n839 = Greater Or Equal?(x=w1115, y=i16 5000) -> (x >= y?=w1123:bool)
                    n840 = Less?(x=w1115, y=i16 5200) -> (x < y?=w1124:bool)
                    n841 = Equal?(x=w1115, y=w1125) -> (x = y?=w1122:bool)
                    n842 = global read "Global.vi" "报警图标"() -> (w1117:refnum<vi>)
                    n843 = And(x=w1123, y=w1124) -> (x .and. y?=w1116:bool)
                    n844 = property class="Bool"(reference=w1117, "Value"=w1116) -> ()  [unwired: 1 in, 2 out]
                    n845 = Bundle By Name(cluster=errorcluster {"status"=FALSE, "code"=0, "source"=""} ("错误常量"), "status"=w1116, "code"=w1115) -> (w1121:errorcluster)
                    n846 = case shown="假" w1122 {
                      tunnel: w1121 -> [w1130 _]
                      frame False {
                        n847 = call "报警处理.vi"("错误常量"=w1130) -> ()  [unwired: 9 in, 2 out]
                      }
                      frame True {
                      }
                    }
                  }
                }
              }
              frame Enabled {
              }
            }
          }
          event User Event {
            n848 = event-data() -> ("试验项"=w1131:T1)  [unwired: 1 in]
            "试验项目" <- w1131
            n849 = disable-structure shown="禁用" {
              disable-tunnel: w1131 -> [w1132 _]
              frame Disabled {
                n850 = global read "A180648.vi" "检测结果"() -> (w1135:string[][][])
                n851 = global read "Global.vi" "Result"() -> (w1133:refnum<vi>)
                n852 = Index Array(array=w1135, index (dim 0)=w1132) -> (element=w1134:string[][])  [unwired: 2 in]
                n853 = property class="Tbl"(reference=w1133, "Value"=w1134) -> ()  [unwired: 1 in, 2 out]
              }
              frame Enabled {
              }
            }
          }
          event "试验项目": Value Change {
            n854 = event-data() -> ("NewVal"=w1136:T1)  [unwired: 1 in]
            n855 = disable-structure shown="禁用" {
              disable-tunnel: w1136 -> [w1140 _]
              frame Disabled {
                n856 = global read "A180648.vi" "检测结果"() -> (w1139:string[][][])
                n857 = global read "Global.vi" "Result"() -> (w1137:refnum<vi>)
                n858 = Index Array(array=w1139, index (dim 0)=w1140) -> (element=w1138:string[][])  [unwired: 2 in]
                n859 = property class="Tbl"(reference=w1137, "Value"=w1138) -> ()  [unwired: 1 in, 2 out]
              }
              frame Enabled {
              }
            }
          }
          event "电流特性试验", "传感器特性试验", "力特性试验", "空载试验", "功能试验", "逆向空载试验", "磨合": Scale Range Change {
            n860 = event-data() -> ("CtlRef"=w1142:refnum<vi>)  [unwired: 1 in, 4 out]
            n861 = global read "Global.vi" "产品型号"() -> (w1141:string)
            n862 = call "XY_conf.vi"("方式"=enum16{"写入", "读取"}."写入", "产品"=w1141, "XY图引用"=w1142) -> ()  [unwired: 4 in, 1 out]
          }
          event User Event {
            n863 = event-data() -> ("产品"=w1145:string)  [unwired: 1 in]
            n864 = control-ref of="传感器特性试验"() -> (w1150:refnum<vi>)
            n865 = control-ref of="逆向空载试验"() -> (w1152:refnum<vi>)
            n866 = control-ref of="电流特性试验"() -> (w1151:refnum<vi>)
            n867 = control-ref of="力特性试验"() -> (w1149:refnum<vi>)
            n868 = control-ref of="磨合"() -> (w1144:refnum<vi>)
            n869 = control-ref of="功能试验"() -> (w1148:refnum<vi>)
            n870 = control-ref of="空载试验"() -> (w1147:refnum<vi>)
            n871 = Build Array(w1152, w1148, w1147, w1151, w1150, w1149, w1144) -> (w1146:refnum<vi>[])
            n872 = for {
              tunnel: w1146 -> [w1154] mode=indexing
              tunnel: w1145 -> [w1153]
              n873 = call "XY_conf.vi"("方式"=enum16{"写入", "读取"}."读取", "产品"=w1153, "XY图引用"=w1154) -> ()  [unwired: 4 in, 1 out]
            }
          }
          event Panel Close {
            n874 = event-data() -> ()  [unwired: 1 in, 4 out]
            n875 = global write "Global.vi" "程序关闭"(TRUE ("程序关闭")) -> ()
          }
          event "电流特性试验", "传感器特性试验", "力特性试验", "空载试验", "功能试验", "逆向空载试验", "磨合": Mouse Enter; "电流特性试验", "传感器特性试验", "力特性试验", "空载试验", "功能试验", "逆向空载试验", "磨合": Mouse Leave; "电流特性试验", "传感器特性试验", "力特性试验", "空载试验", "功能试验", "逆向空载试验": Cursor Move; "磨合": Mouse Move {
            n876 = event-data() -> ("CtlRef"=w1159:refnum<vi>, "Type"=w1157:T25)  [unwired: 1 in]
            n877 = call "CursorShow.vi"("nameShow"=TRUE, "Type"=w1157, "Graph"=w1159) -> ()  [unwired: 7 in, 2 out]
          }
          event "电流特性试验", "传感器特性试验", "力特性试验", "空载试验", "功能试验", "逆向空载试验", "磨合": Mouse Down {
            n878 = event-data() -> ("CtlRef"=w1164:refnum<vi>, "Coords"=w1163:T26, "Type"=w1161:T25)  [unwired: 1 in]
            n879 = invoke class="XYGraph (严格)" method="Map Coords To XY"(reference=w1164, "Coords"=w1163) -> (reference out=w1162:refnum<vi>, "XY"=w1160:cluster{"X":dbl, "Y":dbl})  [unwired: 5 in, 5 out]
            n880 = call "CursorShow.vi"("游标.游标位置"=w1160, "Type"=w1161, "Graph"=w1162) -> ()  [unwired: 7 in, 2 out]
          }
        }
        n881 = global read "Global.vi" "程序关闭"() -> (w1111:bool)
      }
    }
  }
  n882 = Unregister For Events(event registration refnum=w3) -> ()  [unwired: 1 in, 1 out]
